vi "tx poulse host.vi"() -> ()   [LabVIEW 2021]
uses:
  random_limits.ctl
  emitter params.ctl
  mode_type.ctl
  <vilib>/userdefined/High Color/nirio_resource_hc.ctl
  secnario config.ctl
  <instrlib>/niUsrpRio/Config/v1/Host/Public/niUsrpRio Session.ctl
  <instrlib>/_niInstr/Register Bus/v0/Host/Public/Register Bus Session.ctl
  <instrlib>/_niInstr/Register Bus/v0/Host/Private/Session Data.ctl
  <instrlib>/niUsrpRio/Config/v1/Host/Private/DB Queue Reference.ctl
  <instrlib>/niUsrpRio/Config/v1/Host/Private/Daughterboard Data.ctl
  <instrlib>/niUsrpRio/Config/v1/Host/Private/ATR state data.ctl
  <instrlib>/niUsrpRio/Config/v1/Host/Private/Antenna Configuration.ctl
  <instrlib>/niUsrpRio/Config/v1/Host/Private/CPLD Power Mode.ctl
  <instrlib>/niUsrpRio/Config/v1/Host/Public/EEPROM Header.ctl
  <instrlib>/niUsrpRio/Config/v1/Host/Public/EEPROM Device Data Header.ctl
  <instrlib>/niUsrpRio/Config/v1/Host/Public/EEPROM Characterization Header.ctl
  <instrlib>/niUsrpRio/Config/v1/Host/Public/Characterization Data.ctl
  <instrlib>/niUsrpRio/Config/v1/Host/Public/IQ Imbalance.ctl
  <instrlib>/_niInstr/Register Bus/v0/Host/niInstr Register Bus v0 Host.lvlib
  <instrlib>/niUsrpRio/Config/v1/Host/niUsrpRio Config v1 Host.lvlib
panel:
  in  "end program":bool
  in  "Tab Control":T1(tab)=enum."tx configuration"
  in  "user configurations":T3={"vst_device"=["VST_1", "VST_2"], "file paths"=[path "C:/Users/PXIe8108_Demo/Documents/CHAIM DATA/chaim/5785_sync_for_elbit/data/pdw_test_file.tdms", path "C:/Users/PXIe8108_Demo/Documents/CHAIM DATA/chaim/5785_sync_for_elbit/data/pdw_test_file_1.tdms", path "C:/Users/PXIe8108_Demo/Documents/CHAIM DATA/chaim/5785_sync_for_elbit/data/pdw_test_file_2.tdms", path "C:/Users/PXIe8108_Demo/Documents/CHAIM DATA/chaim/5785_sync_for_elbit/data/pdw_test_file_3.tdms", path "C:/Users/PXIe8108_Demo/Documents/CHAIM DATA/chaim/5785_sync_for_elbit/data/pdw_test_file_4.tdms"], "RF gain "=10.0, "devicess "=["IF_transiver_0", "IF_transiver_1", "IF_transiver_2"], "buffer size"=524288, "center frequency (Hz) "=1000000000.0, "Dial"=1, "P2P sample rate"=200000000.0} {"P2P sample rate" format="%#.8p"; "Dial" scale=0.0..3.0; "center frequency (Hz)" format="%#.8p"; "buffer size" step=512; "RF gain" min=-130.0 max=30.0 format="%#.8p"}
  in  "generate":bool
  in  "Tab Control 2":T4(tab)
  in  "rand limits":T5={"DOA range "={1634128.9560392164, 2964508.639841233}, "modulation depth"={67532.40039072247, 205475.5312375231}, "num of hoopers"=25, "num of frequncyes"={2, 1}, "QPSK"=TRUE, "BPSK"=TRUE, "LFM"=TRUE, "CW"=TRUE, "     f band range"={903686635.9447005, 1095391705.0691245}, "D.C range"={0.09831029185867896, 0.026113671274961597}, "hop rate range"={2.0915680786684536, 1602.2122593840786}, "span range "={1634128.9560392164, 2964508.639841233}, "amp range"={-21.121351766513058, -25.88325652841782}, "start time (sec)"=0.0, "end time (sec)"=50.0} {"start time (sec)" format="%#_13g"; "amp range" scale=0.0..-50.0 scale format="%#_g dB"; "span range" scale=1000000.0..3000000000.0 scale format="%#_6p Hz"; "hop rate range" scale=1.0..3000.0 scale format="%#_6p"; "D.C range" scale=0.0..1.0; "f band range" scale=920000000.0..1080000000.0 scale format="%#_6p Hz"; "num of frequncyes" scale=1.0..300.0; "num of hoopers" scale=0.0..200.0; "modulation depth" scale=10000.0..30000000.0 scale format="%#_6p Hz"; "DOA range" scale=0.0..360.0 scale format="%#_6p deg"}
  in  "user bulid emitters":T6[](array[typedef]) {"t end" format="%#_3p"; "t start" format="%#_3p"; "DOA" format="%#_3p"; "mod depth" format="%.0p"}
  in  "convert Button":bool
  in  "csv pulse istraction file in":path=path "C:/Users/PXIe8108_Demo/Documents/CHAIM DATA/chaim/5785_sync_for_elbit/data/pdw_test_file_1.tdms"
  in  "gen for DF":bool=TRUE
  out "num of pulses":i32=902603
  in  "color plate":T8={"PSK Color"=4591, "LFM Color"=15663139, "CW Color"=0}
  in  "refresh_file show":bool
  in  "max number of pulses to show":dbl=500.0
  in  "time range":cluster{dbl, dbl}(slide)={0.0, 78525345.62211981} scale=0.0..50.0 scale format="%#_6p sec"
  out "XY Graph":cluster{dbl[], dbl[]}[](graph)=[{[995507474.9163239, 995507474.9163239, 995394224.6331983, 995394224.6331983, 995507474.9163239], [1.3135e-05, 6.3885e-05, 6.3885e-05, 1.3135e-05, 1.3135e-05]}, {[988830819.370068, 988830819.370068, 988758224.0887612, 988758224.0887612, 988830819.370068], [4.3525e-05, 9.444999999999999e-05, 9.444999999999999e-05, 4.3525e-05, 4.3525e-05]}, {[1062189174.9203769, 1062189174.9203769], [0.000208895, 0.00027960500000000004]}, {[929162452.3956556, 929162452.3956556], [0.00021476, 0.000257185]}, {[1021330874.2578875, 1021330874.2578875], [0.000356845, 0.00040845]}, {[1073135024.1335804, 1073135024.1335804], [0.000418565, 0.000526315]}, {[1060251782.7954887, 1060251782.7954887, 1060128932.6726385, 1060128932.6726385, 1060251782.7954887], [0.000515485, 0.00053533, 0.00053533, 0.000515485, 0.000515485]}, {[1026728042.2238628, 1026728042.2238628], [0.000518575, 0.000544775]}, {[984517369.6351253, 984599401.9622253], [0.000526025, 0.000625825]}, {[992027316.0868192, 992176780.8711365], [0.000643445, 0.00067611]}, {[928917483.6448978, 929054857.2098373], [0.0007013, 0.0007404499999999999]}, {[989419092.0700991, 989419092.0700991, 989346496.7887924, 989346496.7887924, 989419092.0700991], [0.000739625, 0.00079055, 0.00079055, 0.000739625, 0.000739625]}, {[1054560346.3581073, 1054742969.627864], [0.000739975, 0.00084052]}, {[1082291065.6729505, 1082469758.1538203], [0.000779595, 0.00084535]}, {[1050818739.1925838, 1050818739.1925838, 1050641119.2991557, 1050641119.2991557, 1050818739.1925838], [0.000827985, 0.000929745, 0.000929745, 0.000827985, 0.000827985]}, {[1067340749.8623314, 1067340749.8623314, 1067233912.2554936, 1067233912.2554936, 1067340749.8623314], [0.000864145, 0.000954195, 0.000954195, 0.000864145, 0.000864145]}, {[929162452.3956556, 929162452.3956556], [0.001105885, 0.00114831]}, {[996643673.8301789, 996643673.8301789, 996530423.5470532, 996530423.5470532, 996643673.8301789], [0.00112341, 0.00117416, 0.00117416, 0.00112341, 0.00112341]}, {[1082864717.4175386, 1082864717.4175386, 1082774950.8107162, 1082774950.8107162, 1082864717.4175386], [0.001128215, 0.0014517599999999999, 0.0014517599999999999, 0.001128215, 0.001128215]}, {[1031645785.7104015, 1031645785.7104015, 1031564879.5615342, 1031564879.5615342, 1031645785.7104015], [0.00115809, 0.0016224, 0.0016224, 0.00115809, 0.00115809]}, {[1020995471.866172, 1020995471.866172], [0.00117441, 0.001226015]}, {[1062189174.9203769, 1062189174.9203769], [0.001185005, 0.0012557150000000001]}, {[1060210906.3844512, 1060210906.3844512, 1060088056.261601, 1060088056.261601, 1060210906.3844512], [0.001244975, 0.00126482, 0.00126482, 0.001244975, 0.001244975]}, {[1026728042.2238628, 1026728042.2238628], [0.001275565, 0.001301765]}, {[994154871.3947781, 994304336.1790955], [0.00136976, 0.0014024250000000001]}, {[1060103621.4849387, 1060103621.4849387], [0.001372985, 0.0014659949999999999]}, {[988830819.370068, 988830819.370068, 988758224.0887612, 988758224.0887612, 988830819.370068], [0.001435725, 0.00148665, 0.00148665, 0.001435725, 0.001435725]}, {[927476484.2448008, 927613857.8097403], [0.00145419, 0.00149334]}, {[907652360.3992398, 907652360.3992398, 907562914.960957, 907562914.960957, 907652360.3992398], [0.001505205, 0.001655765, 0.001655765, 0.001505205, 0.001505205]}, {[1010524208.2116058, 1010524208.2116058, 1010446688.8317609, 1010446688.8317609, 1010524208.2116058], [0.001643815, 0.0022050100000000003, 0.0022050100000000003, 0.001643815, 0.001643815]}, {[1027479006.2384171, 1027479006.2384171, 1027398361.0771267, 1027398361.0771267, 1027479006.2384171], [0.001671275, 0.0017460800000000001, 0.0017460800000000001, 0.001671275, 0.001671275]}, {[1073152530.0637031, 1073152530.0637031], [0.001702195, 0.001809945]}, {[1080469326.322043, 1080648018.8029127], [0.00176813, 0.001833885]}, {[984517369.6351253, 984599401.9622253], [0.001798725, 0.0018985249999999999]}, {[1055565518.0981148, 1055748141.3678715], [0.001900405, 0.00200095]}, {[1060251782.7954887, 1060251782.7954887, 1060128932.6726385, 1060128932.6726385, 1060251782.7954887], [0.00197447, 0.001994315, 0.001994315, 0.00197447, 0.00197447]}, {[1021330874.2578875, 1021330874.2578875], [0.001991975, 0.00204358]}, {[929162452.3956556, 929162452.3956556], [0.001997015, 0.00203944]}, {[1026728042.2238628, 1026728042.2238628], [0.00203255, 0.0020587500000000002]}, {[992027316.0868192, 992176780.8711365], [0.00209608, 0.002128745]}, {[989419092.0700991, 989419092.0700991, 989346496.7887924, 989346496.7887924, 989419092.0700991], [0.002131825, 0.00218275, 0.00218275, 0.002131825, 0.002131825]}, {[1062189174.9203769, 1062189174.9203769], [0.00216112, 0.0022318299999999998]}, {[928917483.6448978, 929054857.2098373], [0.00220708, 0.00224623]}, {[995507474.9163239, 995507474.9163239, 995394224.6331983, 995394224.6331983, 995507474.9163239], [0.002233685, 0.002284435, 0.002284435, 0.002233685, 0.002233685]}, {[1051290310.7105097, 1051290310.7105097, 1051112690.8170816, 1051112690.8170816, 1051290310.7105097], [0.00251469, 0.00261645, 0.00261645, 0.00251469, 0.00251469]}, {[1060210906.3844512, 1060210906.3844512, 1060088056.261601, 1060088056.261601, 1060210906.3844512], [0.00270396, 0.002723805, 0.002723805, 0.00270396, 0.00270396]}, {[1082291065.6729505, 1082469758.1538203], [0.00275667, 0.002822425]}, {[1026728042.2238628, 1026728042.2238628], [0.00278954, 0.00281574]}, {[1067340749.8623314, 1067340749.8623314, 1067233912.2554936, 1067233912.2554936, 1067340749.8623314], [0.002802505, 0.0028925549999999998, 0.0028925549999999998, 0.002802505, 0.002802505]}, {[1020995471.866172, 1020995471.866172], [0.002809545, 0.0028611500000000002]}, {[994154871.3947781, 994304336.1790955], [0.002822395, 0.00285506]}, {[988830819.370068, 988830819.370068, 988758224.0887612, 988758224.0887612, 988830819.370068], [0.002827925, 0.0028788499999999996, 0.0028788499999999996, 0.002827925, 0.002827925]}, {[929162452.3956556, 929162452.3956556], [0.00288814, 0.002930565]}, {[927476484.2448008, 927613857.8097403], [0.002959975, 0.002999125]}, {[1073135024.1335804, 1073135024.1335804], [0.00298583, 0.0030935800000000003]}, {[1054560346.3581073, 1054742969.627864], [0.00306084, 0.003161385]}, {[984517369.6351253, 984599401.9622253], [0.003071425, 0.003171225]}, {[1062189174.9203769, 1062189174.9203769], [0.00313723, 0.00320794]}, {[959254135.8898987, 959254135.8898987, 959109313.2975742, 959109313.2975742, 959254135.8898987], [0.00317855, 0.00356861, 0.00356861, 0.00317855, 0.00317855]}, {[996643673.8301789, 996643673.8301789, 996530423.5470532, 996530423.5470532, 996643673.8301789], [0.00334396, 0.00339471, 0.00339471, 0.00334396, 0.00334396]}, {[1060251782.7954887, 1060251782.7954887, 1060128932.6726385, 1060128932.6726385, 1060251782.7954887], [0.00343345, 0.003453295, 0.003453295, 0.00343345, 0.00343345]}, {[989419092.0700991, 989419092.0700991, 989346496.7887924, 989346496.7887924, 989419092.0700991], [0.00352402, 0.003574945, 0.003574945, 0.00352402, 0.00352402]}, {[1026728042.2238628, 1026728042.2238628], [0.003546525, 0.003572725]}, {[992027316.0868192, 992176780.8711365], [0.00354871, 0.003581375]}, {[1021330874.2578875, 1021330874.2578875], [0.00362711, 0.003678715]}, {[909232485.1651794, 909232485.1651794, 909143039.7268966, 909143039.7268966, 909232485.1651794], [0.00371271, 0.0038632700000000002, 0.0038632700000000002, 0.00371271, 0.00371271]}, {[928917483.6448978, 929054857.2098373], [0.003712865, 0.003752015]}, {[1080469326.322043, 1080648018.8029127], [0.00374521, 0.003810965]}, {[929162452.3956556, 929162452.3956556], [0.00377927, 0.003821695]}, {[1060103621.4849387, 1060103621.4849387], [0.00394052, 0.0040335300000000004]}, {[1062189174.9203769, 1062189174.9203769], [0.004113345, 0.004184055]}, {[1028479722.7550542, 1028479722.7550542, 1028399077.5937638, 1028399077.5937638, 1028479722.7550542], [0.004155185, 0.0042299899999999994, 0.0042299899999999994, 0.004155185, 0.004155185]}, {[1060210906.3844512, 1060210906.3844512, 1060088056.261601, 1060088056.261601, 1060210906.3844512], [0.00416294, 0.0041827850000000005, 0.0041827850000000005, 0.00416294, 0.00416294]}, {[1050818739.1925838, 1050818739.1925838, 1050641119.2991557, 1050641119.2991557, 1050818739.1925838], [0.00420139, 0.00430315, 0.00430315, 0.00420139, 0.00420139]}, {[988830819.370068, 988830819.370068, 988758224.0887612, 988758224.0887612, 988830819.370068], [0.00422012, 0.004271045, 0.004271045, 0.00422012, 0.00422012]}, {[1055565518.0981148, 1055748141.3678715], [0.00422127, 0.004321815]}, {[1073152530.0637031, 1073152530.0637031], [0.00426946, 0.00437721]}, {[994154871.3947781, 994304336.1790955], [0.00427503, 0.004307695]}, {[1026728042.2238628, 1026728042.2238628], [0.004303515, 0.004329715]}, {[984517369.6351253, 984599401.9622253], [0.004344125, 0.004443925]}, {[1020995471.866172, 1020995471.866172], [0.004444675, 0.00449628]}, {[995507474.9163239, 995507474.9163239, 995394224.6331983, 995394224.6331983, 995507474.9163239], [0.004454235, 0.0045049849999999995, 0.0045049849999999995, 0.004454235, 0.004454235]}, {[927476484.2448008, 927613857.8097403], [0.004465755, 0.004504905]}, {[929162452.3956556, 929162452.3956556], [0.004670395, 0.0047128199999999995]}, {[1083149040.2114863, 1083149040.2114863, 1083059273.6046643, 1083059273.6046643, 1083149040.2114863], [0.00472927, 0.0050528149999999996, 0.0050528149999999996, 0.00472927, 0.00472927]}, {[1082291065.6729505, 1082469758.1538203], [0.004733745, 0.0047995]}, {[1067340749.8623314, 1067340749.8623314, 1067233912.2554936, 1067233912.2554936, 1067340749.8623314], [0.00474086, 0.004830910000000001, 0.004830910000000001, 0.00474086, 0.00474086]}, {[1060251782.7954887, 1060251782.7954887, 1060128932.6726385, 1060128932.6726385, 1060251782.7954887], [0.004892435, 0.00491228, 0.00491228, 0.004892435, 0.004892435]}, {[989419092.0700991, 989419092.0700991, 989346496.7887924, 989346496.7887924, 989419092.0700991], [0.00491622, 0.004967145, 0.004967145, 0.00491622, 0.00491622]}, {[992027316.0868192, 992176780.8711365], [0.005001345, 0.00503401]}, {[1026728042.2238628, 1026728042.2238628], [0.0050605, 0.0050866999999999996]}, {[1062189174.9203769, 1062189174.9203769], [0.005089455, 0.0051601649999999995]}, {[928917483.6448978, 929054857.2098373], [0.005218645, 0.005257795]}, {[958900541.628188, 958900541.628188, 958736338.0157086, 958736338.0157086, 958900541.628188], [0.00525029, 0.00584843, 0.00584843, 0.00525029, 0.00525029]}, {[1021330874.2578875, 1021330874.2578875], [0.00526224, 0.005313844999999999]}, {[1054560346.3581073, 1054742969.627864], [0.005381705, 0.005482249999999999]}, {[1073135024.1335804, 1073135024.1335804], [0.005553095, 0.005660845]}, {[929162452.3956556, 929162452.3956556], [0.00556152, 0.005603945]}, {[996643673.8301789, 996643673.8301789, 996530423.5470532, 996530423.5470532, 996643673.8301789], [0.005564505, 0.0056152549999999996, 0.0056152549999999996, 0.005564505, 0.005564505]}, {[988830819.370068, 988830819.370068, 988758224.0887612, 988758224.0887612, 988830819.370068], [0.00561232, 0.005663245, 0.005663245, 0.00561232, 0.00561232]}, {[984517369.6351253, 984599401.9622253], [0.005616825, 0.0057166249999999995]}, {[1060210906.3844512, 1060210906.3844512, 1060088056.261601, 1060088056.261601, 1060210906.3844512], [0.005621925, 0.00564177, 0.00564177, 0.005621925, 0.005621925]}, {[1080469326.322043, 1080648018.8029127], [0.005722285, 0.0057880399999999995]}, {[994154871.3947781, 994304336.1790955], [0.00572766, 0.005760325]}, {[1026728042.2238628, 1026728042.2238628], [0.00581749, 0.0058436899999999995]}, {[1051290310.7105097, 1051290310.7105097, 1051112690.8170816, 1051112690.8170816, 1051290310.7105097], [0.005888095, 0.0059898550000000005, 0.0059898550000000005, 0.005888095, 0.005888095]}, {[907652360.3992398, 907652360.3992398, 907562914.960957, 907562914.960957, 907652360.3992398], [0.005920215, 0.0060707750000000005, 0.0060707750000000005, 0.005920215, 0.005920215]}, {[927476484.2448008, 927613857.8097403], [0.005971535, 0.006010685]}, {[1062189174.9203769, 1062189174.9203769], [0.00606557, 0.00613628]}, {[1020995471.866172, 1020995471.866172], [0.00607981, 0.0061314149999999994]}, {[989419092.0700991, 989419092.0700991, 989346496.7887924, 989346496.7887924, 989419092.0700991], [0.006308415, 0.006359340000000001, 0.006359340000000001, 0.006308415, 0.006308415]}, {[1060251782.7954887, 1060251782.7954887, 1060128932.6726385, 1060128932.6726385, 1060251782.7954887], [0.006351415, 0.00637126, 0.00637126, 0.006351415, 0.006351415]}, {[1032360862.9064839, 1032360862.9064839, 1032279956.7576165, 1032279956.7576165, 1032360862.9064839], [0.006364295, 0.006828605, 0.006828605, 0.006364295, 0.006364295]}, {[929162452.3956556, 929162452.3956556], [0.00645265, 0.0064950749999999995]}, {[992027316.0868192, 992176780.8711365], [0.00645398, 0.006486645]}, {[1060103621.4849387, 1060103621.4849387], [0.00650806, 0.0066010700000000005]}, {[1055565518.0981148, 1055748141.3678715], [0.006542135, 0.00664268]}, {[1026728042.2238628, 1026728042.2238628], [0.00657448, 0.006600679999999999]}, {[1027479006.2384171, 1027479006.2384171, 1027398361.0771267, 1027398361.0771267, 1027479006.2384171], [0.006639095, 0.0067139, 0.0067139, 0.006639095, 0.006639095]}, {[995507474.9163239, 995507474.9163239, 995394224.6331983, 995394224.6331983, 995507474.9163239], [0.00667478, 0.0067255299999999995, 0.0067255299999999995, 0.00667478, 0.00667478]}, {[1067340749.8623314, 1067340749.8623314, 1067233912.2554936, 1067233912.2554936, 1067340749.8623314], [0.00667922, 0.00676927, 0.00676927, 0.00667922, 0.00667922]}, {[1082291065.6729505, 1082469758.1538203], [0.006710825, 0.00677658]}, {[928917483.6448978, 929054857.2098373], [0.006724425, 0.006763575]}, {[1073152530.0637031, 1073152530.0637031], [0.00683673, 0.00694448]}, {[984517369.6351253, 984599401.9622253], [0.006889525, 0.006989324999999999]}, {[1021330874.2578875, 1021330874.2578875], [0.006897375, 0.00694898]}, {[988830819.370068, 988830819.370068, 988758224.0887612, 988758224.0887612, 988830819.370068], [0.007004515, 0.0070554400000000005, 0.0070554400000000005, 0.007004515, 0.007004515]}, {[1062189174.9203769, 1062189174.9203769], [0.00704168, 0.00711239]}, {[1060210906.3844512, 1060210906.3844512, 1060088056.261601, 1060088056.261601, 1060210906.3844512], [0.007080905, 0.00710075, 0.00710075, 0.007080905, 0.007080905]}, {[994154871.3947781, 994304336.1790955], [0.007180295, 0.00721296]}, {[1026728042.2238628, 1026728042.2238628], [0.007331465, 0.007357664999999999]}, {[929162452.3956556, 929162452.3956556], [0.007343775, 0.0073862]}, {[927476484.2448008, 927613857.8097403], [0.00747732, 0.00751647]}, {[1050818739.1925838, 1050818739.1925838, 1050641119.2991557, 1050641119.2991557, 1050818739.1925838], [0.0075748, 0.00767656, 0.00767656, 0.0075748, 0.0075748]}, {[959254135.8898987, 959254135.8898987, 959109313.2975742, 959109313.2975742, 959254135.8898987], [0.00769425, 0.008084309999999999, 0.008084309999999999, 0.00769425, 0.00769425]}, {[1080469326.322043, 1080648018.8029127], [0.00769936, 0.0077651149999999995]}, {[989419092.0700991, 989419092.0700991, 989346496.7887924, 989346496.7887924, 989419092.0700991], [0.007700615, 0.00775154, 0.00775154, 0.007700615, 0.007700615]}, {[1054560346.3581073, 1054742969.627864], [0.00770257, 0.007803114999999999]}, {[1020995471.866172, 1020995471.866172], [0.00771494, 0.007766545]}, {[996643673.8301789, 996643673.8301789, 996530423.5470532, 996530423.5470532, 996643673.8301789], [0.007785055, 0.007835805, 0.007835805, 0.007785055, 0.007785055]}, {[1060251782.7954887, 1060251782.7954887, 1060128932.6726385, 1060128932.6726385, 1060251782.7954887], [0.0078104, 0.007830245, 0.007830245, 0.0078104, 0.0078104]}, {[992027316.0868192, 992176780.8711365], [0.00790661, 0.007939274999999999]}, {[1062189174.9203769, 1062189174.9203769], [0.008017795, 0.008088505]}, {[1010524208.2116058, 1010524208.2116058, 1010446688.8317609, 1010446688.8317609, 1010524208.2116058], [0.008022065, 0.00858326, 0.00858326, 0.008022065, 0.008022065]}, {[1026728042.2238628, 1026728042.2238628], [0.008088455, 0.008114655]}, {[1073135024.1335804, 1073135024.1335804], [0.00812036, 0.00822811]}, {[909232485.1651794, 909232485.1651794, 909143039.7268966, 909143039.7268966, 909232485.1651794], [0.00812772, 0.008278279999999999, 0.008278279999999999, 0.00812772, 0.00812772]}, {[984517369.6351253, 984599401.9622253], [0.008162225, 0.008262025000000001]}, {[928917483.6448978, 929054857.2098373], [0.00823021, 0.00826936]}, {[929162452.3956556, 929162452.3956556], [0.0082349, 0.008277325]}, {[1082864717.4175386, 1082864717.4175386, 1082774950.8107162, 1082774950.8107162, 1082864717.4175386], [0.00833032, 0.008653865, 0.008653865, 0.00833032, 0.00833032]}, {[988830819.370068, 988830819.370068, 988758224.0887612, 988758224.0887612, 988830819.370068], [0.008396715, 0.008447640000000001, 0.008447640000000001, 0.008396715, 0.008396715]}, {[1021330874.2578875, 1021330874.2578875], [0.008532505, 0.008584109999999999]}, {[1060210906.3844512, 1060210906.3844512, 1060088056.261601, 1060088056.261601, 1060210906.3844512], [0.00853989, 0.008559734999999999, 0.008559734999999999, 0.00853989, 0.00853989]}, {[1067340749.8623314, 1067340749.8623314, 1067233912.2554936, 1067233912.2554936, 1067340749.8623314], [0.00861758, 0.00870763, 0.00870763, 0.00861758, 0.00861758]}, {[994154871.3947781, 994304336.1790955], [0.00863293, 0.008665595]}, {[1082291065.6729505, 1082469758.1538203], [0.0086879, 0.008753655]}, {[1026728042.2238628, 1026728042.2238628], [0.00884544, 0.00887164]}, {[1055565518.0981148, 1055748141.3678715], [0.008863, 0.008963545]}, {[1071939451.6053249, 1071939451.6053249, 1071769816.3211857, 1071769816.3211857, 1071939451.6053249], [0.008890785, 0.009210155, 0.009210155, 0.008890785, 0.008890785]}, {[995507474.9163239, 995507474.9163239, 995394224.6331983, 995394224.6331983, 995507474.9163239], [0.00889533, 0.00894608, 0.00894608, 0.00889533, 0.00889533]}, {[920932748.9465165, 920932748.9465165, 920784710.4565091, 920784710.4565091, 920932748.9465165], [0.00893469, 0.009550165000000001, 0.009550165000000001, 0.00893469, 0.00893469]}, {[927476484.2448008, 927613857.8097403], [0.0089831, 0.00902225]}, {[1062189174.9203769, 1062189174.9203769], [0.008993905, 0.009064615]}, {[1060103621.4849387, 1060103621.4849387], [0.009075595, 0.009168605]}, {[989419092.0700991, 989419092.0700991, 989346496.7887924, 989346496.7887924, 989419092.0700991], [0.009092815, 0.009143740000000001, 0.009143740000000001, 0.009092815, 0.009092815]}, {[1028479722.7550542, 1028479722.7550542, 1028399077.5937638, 1028399077.5937638, 1028479722.7550542], [0.009123005, 0.00919781, 0.00919781, 0.009123005, 0.009123005]}, {[929162452.3956556, 929162452.3956556], [0.00912603, 0.009168455]}, {[1051290310.7105097, 1051290310.7105097, 1051112690.8170816, 1051112690.8170816, 1051290310.7105097], [0.009261505, 0.009363264999999999, 0.009363264999999999, 0.009261505, 0.009261505]}, {[1060251782.7954887, 1060251782.7954887, 1060128932.6726385, 1060128932.6726385, 1060251782.7954887], [0.00926938, 0.009289225, 0.009289225, 0.00926938, 0.00926938]}, {[1020995471.866172, 1020995471.866172], [0.009350075, 0.009401679999999999]}, {[992027316.0868192, 992176780.8711365], [0.009359245, 0.00939191]}, {[1073152530.0637031, 1073152530.0637031], [0.009403995, 0.009511745]}, {[984517369.6351253, 984599401.9622253], [0.009434925, 0.009534725]}, {[1026728042.2238628, 1026728042.2238628], [0.00960243, 0.009628630000000001]}, {[1080469326.322043, 1080648018.8029127], [0.009676435, 0.009742190000000001]}, {[928917483.6448978, 929054857.2098373], [0.00973599, 0.00977514]}, {[988830819.370068, 988830819.370068, 988758224.0887612, 988758224.0887612, 988830819.370068], [0.00978891, 0.009839835, 0.009839835, 0.00978891, 0.00978891]}, {[1062189174.9203769, 1062189174.9203769], [0.00997002, 0.01004073]}, {[1060210906.3844512, 1060210906.3844512, 1060088056.261601, 1060088056.261601, 1060210906.3844512], [0.00999887, 0.010018715, 0.010018715, 0.00999887, 0.00999887]}, {[996643673.8301789, 996643673.8301789, 996530423.5470532, 996530423.5470532, 996643673.8301789], [0.010005605, 0.010056355000000001, 0.010056355000000001, 0.010005605, 0.010005605]}, {[929162452.3956556, 929162452.3956556], [0.010017155, 0.01005958]}, {[1054560346.3581073, 1054742969.627864], [0.010023435, 0.010123980000000001]}, {[994154871.3947781, 994304336.1790955], [0.01008556, 0.010118225]}, {[1021330874.2578875, 1021330874.2578875], [0.01016764, 0.010219245]}, {[907652360.3992398, 907652360.3992398, 907562914.960957, 907562914.960957, 907652360.3992398], [0.010335225, 0.010485785, 0.010485785, 0.010335225, 0.010335225]}, {[1026728042.2238628, 1026728042.2238628], [0.010359415, 0.010385615]}, {[989419092.0700991, 989419092.0700991, 989346496.7887924, 989346496.7887924, 989419092.0700991], [0.01048501, 0.010535935, 0.010535935, 0.01048501, 0.01048501]}, {[927476484.2448008, 927613857.8097403], [0.01048888, 0.01052803]}, {[1067340749.8623314, 1067340749.8623314, 1067233912.2554936, 1067233912.2554936, 1067340749.8623314], [0.010555935, 0.010645985, 0.010645985, 0.010555935, 0.010555935]}, {[1082291065.6729505, 1082469758.1538203], [0.010664975, 0.01073073]}, {[1073135024.1335804, 1073135024.1335804], [0.010687625, 0.010795375]}, {[984517369.6351253, 984599401.9622253], [0.010707625, 0.010807425]}, {[1060251782.7954887, 1060251782.7954887, 1060128932.6726385, 1060128932.6726385, 1060251782.7954887], [0.01072836, 0.010748204999999999, 0.010748204999999999, 0.01072836, 0.01072836]}, {[992027316.0868192, 992176780.8711365], [0.01081188, 0.010844544999999999]}, {[929162452.3956556, 929162452.3956556], [0.01090828, 0.010950705]}, {[1062189174.9203769, 1062189174.9203769], [0.01094613, 0.01101684]}, {[1050818739.1925838, 1050818739.1925838, 1050641119.2991557, 1050641119.2991557, 1050818739.1925838], [0.01094821, 0.01104997, 0.01104997, 0.01094821, 0.01094821]}, {[1020995471.866172, 1020995471.866172], [0.010985205, 0.01103681]}, {[995507474.9163239, 995507474.9163239, 995394224.6331983, 995394224.6331983, 995507474.9163239], [0.01111588, 0.01116663, 0.01116663, 0.01111588, 0.01111588]}, {[1026728042.2238628, 1026728042.2238628], [0.011116405, 0.011142605]}, {[988830819.370068, 988830819.370068, 988758224.0887612, 988758224.0887612, 988830819.370068], [0.01118111, 0.011232035, 0.011232035, 0.01118111, 0.01118111]}, {[1055565518.0981148, 1055748141.3678715], [0.011183865, 0.01128441]}, {[928917483.6448978, 929054857.2098373], [0.011241775, 0.011280925]}, {[1060210906.3844512, 1060210906.3844512, 1060088056.261601, 1060088056.261601, 1060210906.3844512], [0.011457855, 0.011477699999999999, 0.011477699999999999, 0.011457855, 0.011457855]}, {[994154871.3947781, 994304336.1790955], [0.011538195, 0.011570859999999999]}, {[1031645785.7104015, 1031645785.7104015, 1031564879.5615342, 1031564879.5615342, 1031645785.7104015], [0.011570505, 0.012034815, 0.012034815, 0.011570505, 0.011570505]}, {[1027479006.2384171, 1027479006.2384171, 1027398361.0771267, 1027398361.0771267, 1027479006.2384171], [0.011606915, 0.011681720000000001, 0.011681720000000001, 0.011606915, 0.011606915]}, {[1060103621.4849387, 1060103621.4849387], [0.01164313, 0.011736139999999999]}, {[1080469326.322043, 1080648018.8029127], [0.011653515, 0.01171927]}, {[929162452.3956556, 929162452.3956556], [0.01179941, 0.011841835]}, {[1021330874.2578875, 1021330874.2578875], [0.01180277, 0.011854375]}, {[1026728042.2238628, 1026728042.2238628], [0.011873395, 0.011899595]}, {[989419092.0700991, 989419092.0700991, 989346496.7887924, 989346496.7887924, 989419092.0700991], [0.01187721, 0.011928135, 0.011928135, 0.01187721, 0.01187721]}, {[1062189174.9203769, 1062189174.9203769], [0.011922245, 0.011992955]}, {[1083149040.2114863, 1083149040.2114863, 1083059273.6046643, 1083059273.6046643, 1083149040.2114863], [0.01193137, 0.012254915, 0.012254915, 0.01193137, 0.01193137]}, {[1073152530.0637031, 1073152530.0637031], [0.01197126, 0.01207901]}, {[984517369.6351253, 984599401.9622253], [0.011980325, 0.012080125]}, {[927476484.2448008, 927613857.8097403], [0.011994665, 0.012033815]}, {[1060251782.7954887, 1060251782.7954887, 1060128932.6726385, 1060128932.6726385, 1060251782.7954887], [0.012187345, 0.01220719, 0.01220719, 0.012187345, 0.012187345]}, {[959254135.8898987, 959254135.8898987, 959109313.2975742, 959109313.2975742, 959254135.8898987], [0.01220995, 0.01260001, 0.01260001, 0.01220995, 0.01220995]}, {[996643673.8301789, 996643673.8301789, 996530423.5470532, 996530423.5470532, 996643673.8301789], [0.01222615, 0.0122769, 0.0122769, 0.01222615, 0.01222615]}, {[992027316.0868192, 992176780.8711365], [0.01226451, 0.012297174999999999]}, {[1054560346.3581073, 1054742969.627864], [0.012344295, 0.01244484]}, {[1067340749.8623314, 1067340749.8623314, 1067233912.2554936, 1067233912.2554936, 1067340749.8623314], [0.012494295, 0.012584345, 0.012584345, 0.012494295, 0.012494295]}, {[909232485.1651794, 909232485.1651794, 909143039.7268966, 909143039.7268966, 909232485.1651794], [0.01254273, 0.01269329, 0.01269329, 0.01254273, 0.01254273]}, {[988830819.370068, 988830819.370068, 988758224.0887612, 988758224.0887612, 988830819.370068], [0.01257331, 0.012624235000000001, 0.012624235000000001, 0.01257331, 0.01257331]}, {[1020995471.866172, 1020995471.866172], [0.01262034, 0.012671945]}, {[1026728042.2238628, 1026728042.2238628], [0.01263038, 0.01265658]}, {[1051290310.7105097, 1051290310.7105097, 1051112690.8170816, 1051112690.8170816, 1051290310.7105097], [0.01263491, 0.012736669999999999, 0.012736669999999999, 0.01263491, 0.01263491]}, {[1082291065.6729505, 1082469758.1538203], [0.01264205, 0.012707805]}, {[929162452.3956556, 929162452.3956556], [0.012690535, 0.01273296]}, {[928917483.6448978, 929054857.2098373], [0.012747555, 0.012786705]}, {[1062189174.9203769, 1062189174.9203769], [0.012898355, 0.012969065]}, {[1060210906.3844512, 1060210906.3844512, 1060088056.261601, 1060088056.261601, 1060210906.3844512], [0.012916835, 0.012936679999999999, 0.012936679999999999, 0.012916835, 0.012916835]}, {[958900541.628188, 958900541.628188, 958736338.0157086, 958736338.0157086, 958900541.628188], [0.01294312, 0.013541260000000001, 0.013541260000000001, 0.01294312, 0.01294312]}, {[994154871.3947781, 994304336.1790955], [0.01299083, 0.013023495]}, {[984517369.6351253, 984599401.9622253], [0.013253025, 0.013352825]}, {[1073135024.1335804, 1073135024.1335804], [0.01325489, 0.01336264]}, {[989419092.0700991, 989419092.0700991, 989346496.7887924, 989346496.7887924, 989419092.0700991], [0.013269405, 0.01332033, 0.01332033, 0.013269405, 0.013269405]}, {[995507474.9163239, 995507474.9163239, 995394224.6331983, 995394224.6331983, 995507474.9163239], [0.013336425, 0.013387175000000001, 0.013387175000000001, 0.013336425, 0.013336425]}, {[1026728042.2238628, 1026728042.2238628], [0.01338737, 0.013413570000000001]}, {[1021330874.2578875, 1021330874.2578875], [0.013437905, 0.01348951]}, {[927476484.2448008, 927613857.8097403], [0.013500445, 0.013539595]}, {[1055565518.0981148, 1055748141.3678715], [0.01350473, 0.013605275]}, {[929162452.3956556, 929162452.3956556], [0.013581665, 0.01362409]}, {[1080469326.322043, 1080648018.8029127], [0.01363059, 0.013696345]}, {[1060251782.7954887, 1060251782.7954887, 1060128932.6726385, 1060128932.6726385, 1060251782.7954887], [0.013646325, 0.01366617, 0.01366617, 0.013646325, 0.013646325]}, {[992027316.0868192, 992176780.8711365], [0.013717145, 0.01374981]}, {[1062189174.9203769, 1062189174.9203769], [0.01387447, 0.01394518]}, {[988830819.370068, 988830819.370068, 988758224.0887612, 988758224.0887612, 988830819.370068], [0.013965505, 0.01401643, 0.01401643, 0.013965505, 0.013965505]}, {[1028479722.7550542, 1028479722.7550542, 1028399077.5937638, 1028399077.5937638, 1028479722.7550542], [0.014090825, 0.01416563, 0.01416563, 0.014090825, 0.014090825]}, {[1026728042.2238628, 1026728042.2238628], [0.014144355, 0.014170555000000001]}, {[1060103621.4849387, 1060103621.4849387], [0.01421067, 0.01430368]}, {[928917483.6448978, 929054857.2098373], [0.014253335, 0.014292485]}, {[1020995471.866172, 1020995471.866172], [0.01425547, 0.014307074999999999]}, {[1050818739.1925838, 1050818739.1925838, 1050641119.2991557, 1050641119.2991557, 1050818739.1925838], [0.014321615, 0.014423374999999999, 0.014423374999999999, 0.014321615, 0.014321615]}, {[1060210906.3844512, 1060210906.3844512, 1060088056.261601, 1060088056.261601, 1060210906.3844512], [0.01437582, 0.014395664999999998, 0.014395664999999998, 0.01437582, 0.01437582]}, {[1010524208.2116058, 1010524208.2116058, 1010446688.8317609, 1010446688.8317609, 1010524208.2116058], [0.01440032, 0.014961515, 0.014961515, 0.01440032, 0.01440032]}, {[1067340749.8623314, 1067340749.8623314, 1067233912.2554936, 1067233912.2554936, 1067340749.8623314], [0.014432655, 0.014522705, 0.014522705, 0.014432655, 0.014432655]}, {[994154871.3947781, 994304336.1790955], [0.01444346, 0.014476125]}, {[996643673.8301789, 996643673.8301789, 996530423.5470532, 996530423.5470532, 996643673.8301789], [0.0144467, 0.01449745, 0.01449745, 0.0144467, 0.0144467]}, {[929162452.3956556, 929162452.3956556], [0.01447279, 0.014515215]}, {[984517369.6351253, 984599401.9622253], [0.01452572, 0.014625520000000001]}, {[1073152530.0637031, 1073152530.0637031], [0.014538525, 0.014646275]}, {[1082291065.6729505, 1082469758.1538203], [0.01461913, 0.014684885]}, {[989419092.0700991, 989419092.0700991, 989346496.7887924, 989346496.7887924, 989419092.0700991], [0.014661605, 0.01471253, 0.01471253, 0.014661605, 0.014661605]}, {[1054560346.3581073, 1054742969.627864], [0.01466516, 0.014765705]}, {[907652360.3992398, 907652360.3992398, 907562914.960957, 907562914.960957, 907652360.3992398], [0.014750235, 0.014900795, 0.014900795, 0.014750235, 0.014750235]}, {[1062189174.9203769, 1062189174.9203769], [0.01485058, 0.01492129]}, {[1026728042.2238628, 1026728042.2238628], [0.014901345, 0.014927545]}, {[927476484.2448008, 927613857.8097403], [0.015006225, 0.015045375]}, {[1021330874.2578875, 1021330874.2578875], [0.015073035, 0.01512464]}, {[1060251782.7954887, 1060251782.7954887, 1060128932.6726385, 1060128932.6726385, 1060251782.7954887], [0.01510531, 0.015125155, 0.015125155, 0.01510531, 0.01510531]}, {[992027316.0868192, 992176780.8711365], [0.01516978, 0.015202445]}, {[988830819.370068, 988830819.370068, 988758224.0887612, 988758224.0887612, 988830819.370068], [0.015357705, 0.01540863, 0.01540863, 0.015357705, 0.015357705]}, {[929162452.3956556, 929162452.3956556], [0.015363915, 0.015406340000000001]}, {[1082864717.4175386, 1082864717.4175386, 1082774950.8107162, 1082774950.8107162, 1082864717.4175386], [0.015532425, 0.01585597, 0.01585597, 0.015532425, 0.015532425]}, {[995507474.9163239, 995507474.9163239, 995394224.6331983, 995394224.6331983, 995507474.9163239], [0.015556975, 0.015607725000000001, 0.015607725000000001, 0.015556975, 0.015556975]}, {[1080469326.322043, 1080648018.8029127], [0.015607665, 0.01567342]}, {[1026728042.2238628, 1026728042.2238628], [0.01565833, 0.015684530000000002]}, {[928917483.6448978, 929054857.2098373], [0.01575912, 0.015798270000000003]}, {[984517369.6351253, 984599401.9622253], [0.01579842, 0.01589822]}, {[1073135024.1335804, 1073135024.1335804], [0.015822155, 0.015929905]}, {[1055565518.0981148, 1055748141.3678715], [0.015825595, 0.015926140000000002]}, {[1062189174.9203769, 1062189174.9203769], [0.015826695, 0.015897405000000003]}, {[1060210906.3844512, 1060210906.3844512, 1060088056.261601, 1060088056.261601, 1060210906.3844512], [0.0158348, 0.015854645, 0.015854645, 0.0158348, 0.0158348]}, {[1020995471.866172, 1020995471.866172], [0.015890605, 0.01594221]}, {[994154871.3947781, 994304336.1790955], [0.015896095, 0.01592876]}, {[1051290310.7105097, 1051290310.7105097, 1051112690.8170816, 1051112690.8170816, 1051290310.7105097], [0.01600832, 0.01611008, 0.01611008, 0.01600832, 0.01600832]}, {[989419092.0700991, 989419092.0700991, 989346496.7887924, 989346496.7887924, 989419092.0700991], [0.0160538, 0.016104725, 0.016104725, 0.0160538, 0.0160538]}, {[929162452.3956556, 929162452.3956556], [0.016255045, 0.016297469999999998]}, {[1067340749.8623314, 1067340749.8623314, 1067233912.2554936, 1067233912.2554936, 1067340749.8623314], [0.016371015, 0.016461065, 0.016461065, 0.016371015, 0.016371015]}, {[1026728042.2238628, 1026728042.2238628], [0.01641532, 0.01644152]}, {[927476484.2448008, 927613857.8097403], [0.01651201, 0.016551160000000002]}, {[1060251782.7954887, 1060251782.7954887, 1060128932.6726385, 1060128932.6726385, 1060251782.7954887], [0.01656429, 0.016584135, 0.016584135, 0.01656429, 0.01656429]}, {[1027479006.2384171, 1027479006.2384171, 1027398361.0771267, 1027398361.0771267, 1027479006.2384171], [0.016574735, 0.01664954, 0.01664954, 0.016574735, 0.016574735]}, {[1082291065.6729505, 1082469758.1538203], [0.016596205, 0.01666196]}, {[992027316.0868192, 992176780.8711365], [0.01662241, 0.016655075000000002]}, {[996643673.8301789, 996643673.8301789, 996530423.5470532, 996530423.5470532, 996643673.8301789], [0.01666725, 0.016718, 0.016718, 0.01666725, 0.01666725]}, {[1021330874.2578875, 1021330874.2578875], [0.01670817, 0.016759775]}, {[959254135.8898987, 959254135.8898987, 959109313.2975742, 959109313.2975742, 959254135.8898987], [0.01672565, 0.017115710000000003, 0.017115710000000003, 0.01672565, 0.01672565]}, {[988830819.370068, 988830819.370068, 988758224.0887612, 988758224.0887612, 988830819.370068], [0.0167499, 0.016800825000000002, 0.016800825000000002, 0.0167499, 0.0167499]}, {[1032360862.9064839, 1032360862.9064839, 1032279956.7576165, 1032279956.7576165, 1032360862.9064839], [0.01677671, 0.01724102, 0.01724102, 0.01677671, 0.01677671]}, {[1060103621.4849387, 1060103621.4849387], [0.016778205, 0.016871215000000002]}, {[1062189174.9203769, 1062189174.9203769], [0.016802805, 0.016873515000000002]}, {[909232485.1651794, 909232485.1651794, 909143039.7268966, 909143039.7268966, 909232485.1651794], [0.016957735, 0.017108295000000003, 0.017108295000000003, 0.016957735, 0.016957735]}, {[1054560346.3581073, 1054742969.627864], [0.016986025, 0.01708657]}, {[984517369.6351253, 984599401.9622253], [0.01707112, 0.01717092]}, {[1073152530.0637031, 1073152530.0637031], [0.01710579, 0.01721354]}, {[929162452.3956556, 929162452.3956556], [0.01714617, 0.017188594999999997]}, {[1026728042.2238628, 1026728042.2238628], [0.017172305, 0.017198505]}, {[928917483.6448978, 929054857.2098373], [0.0172649, 0.01730405]}, {[1060210906.3844512, 1060210906.3844512, 1060088056.261601, 1060088056.261601, 1060210906.3844512], [0.017293785, 0.01731363, 0.01731363, 0.017293785, 0.017293785]}, {[994154871.3947781, 994304336.1790955], [0.017348725, 0.01738139]}, {[989419092.0700991, 989419092.0700991, 989346496.7887924, 989346496.7887924, 989419092.0700991], [0.017446, 0.017496925, 0.017496925, 0.017446, 0.017446]}, {[1020995471.866172, 1020995471.866172], [0.017525735, 0.01757734]}, {[1080469326.322043, 1080648018.8029127], [0.017584745, 0.0176505]}, {[1050818739.1925838, 1050818739.1925838, 1050641119.2991557, 1050641119.2991557, 1050818739.1925838], [0.017695025, 0.017796785, 0.017796785, 0.017695025, 0.017695025]}, {[995507474.9163239, 995507474.9163239, 995394224.6331983, 995394224.6331983, 995507474.9163239], [0.017777525, 0.017828274999999998, 0.017828274999999998, 0.017777525, 0.017777525]}, {[1062189174.9203769, 1062189174.9203769], [0.01777892, 0.017849630000000002]}, {[1069922913.2514993, 1069922913.2514993, 1069753277.9673601, 1069753277.9673601, 1069922913.2514993], [0.01780574, 0.01812511, 0.01812511, 0.01780574, 0.01780574]}, {[1026728042.2238628, 1026728042.2238628], [0.017929295, 0.017955495000000002]}, {[927476484.2448008, 927613857.8097403], [0.01801779, 0.01805694]}, {[1060251782.7954887, 1060251782.7954887, 1060128932.6726385, 1060128932.6726385, 1060251782.7954887], [0.018023275, 0.01804312, 0.01804312, 0.018023275, 0.018023275]}, {[929162452.3956556, 929162452.3956556], [0.018037295, 0.018079719999999997]}, {[992027316.0868192, 992176780.8711365], [0.018075045, 0.018107710000000003]}, {[988830819.370068, 988830819.370068, 988758224.0887612, 988758224.0887612, 988830819.370068], [0.0181421, 0.018193025, 0.018193025, 0.0181421, 0.0181421]}, {[1055565518.0981148, 1055748141.3678715], [0.01814646, 0.018247005]}, {[1067340749.8623314, 1067340749.8623314, 1067233912.2554936, 1067233912.2554936, 1067340749.8623314], [0.01830937, 0.01839942, 0.01839942, 0.01830937, 0.01830937]}, {[1021330874.2578875, 1021330874.2578875], [0.0183433, 0.018394905]}, {[984517369.6351253, 984599401.9622253], [0.01834382, 0.01844362]}, {[1073135024.1335804, 1073135024.1335804], [0.01838942, 0.01849717]}, {[1082291065.6729505, 1082469758.1538203], [0.01857328, 0.018639035]}, {[1026728042.2238628, 1026728042.2238628], [0.018686285, 0.018712485]}, {[1060210906.3844512, 1060210906.3844512, 1060088056.261601, 1060088056.261601, 1060210906.3844512], [0.018752765, 0.018772610000000002, 0.018772610000000002, 0.018752765, 0.018752765]}, {[1062189174.9203769, 1062189174.9203769], [0.01875503, 0.01882574]}, {[928917483.6448978, 929054857.2098373], [0.01877068, 0.018809830000000003]}, {[994154871.3947781, 994304336.1790955], [0.01880136, 0.018834025]}, {[989419092.0700991, 989419092.0700991, 989346496.7887924, 989346496.7887924, 989419092.0700991], [0.0188382, 0.018889125, 0.018889125, 0.0188382, 0.0188382]}, {[996643673.8301789, 996643673.8301789, 996530423.5470532, 996530423.5470532, 996643673.8301789], [0.018887795, 0.018938544999999998, 0.018938544999999998, 0.018887795, 0.018887795]}, {[929162452.3956556, 929162452.3956556], [0.018928425, 0.018970849999999997]}, {[1028479722.7550542, 1028479722.7550542, 1028399077.5937638, 1028399077.5937638, 1028479722.7550542], [0.01905864, 0.019133445000000002, 0.019133445000000002, 0.01905864, 0.01905864]}, {[1083149040.2114863, 1083149040.2114863, 1083059273.6046643, 1083059273.6046643, 1083149040.2114863], [0.019133475, 0.019457020000000002, 0.019457020000000002, 0.019133475, 0.019133475]}, {[1020995471.866172, 1020995471.866172], [0.01916087, 0.019212475]}, {[907652360.3992398, 907652360.3992398, 907562914.960957, 907562914.960957, 907652360.3992398], [0.01916524, 0.0193158, 0.0193158, 0.01916524, 0.01916524]}, {[1054560346.3581073, 1054742969.627864], [0.01930689, 0.019407435]}, {[1060103621.4849387, 1060103621.4849387], [0.019345745, 0.019438755000000002]}, {[1051290310.7105097, 1051290310.7105097, 1051112690.8170816, 1051112690.8170816, 1051290310.7105097], [0.019381725, 0.019483485, 0.019483485, 0.019381725, 0.019381725]}, {[1026728042.2238628, 1026728042.2238628], [0.01944327, 0.01946947]}, {[1060251782.7954887, 1060251782.7954887, 1060128932.6726385, 1060128932.6726385, 1060251782.7954887], [0.019482255, 0.0195021, 0.0195021, 0.019482255, 0.019482255]}, {[927476484.2448008, 927613857.8097403], [0.019523575, 0.019562725000000003]}, {[992027316.0868192, 992176780.8711365], [0.019527675, 0.019560340000000002]}, {[988830819.370068, 988830819.370068, 988758224.0887612, 988758224.0887612, 988830819.370068], [0.019534295, 0.01958522, 0.01958522, 0.019534295, 0.019534295]}, {[1080469326.322043, 1080648018.8029127], [0.01956182, 0.019627575]}, {[984517369.6351253, 984599401.9622253], [0.01961652, 0.01971632]}, {[1073152530.0637031, 1073152530.0637031], [0.019673055, 0.019780805]}, {[1062189174.9203769, 1062189174.9203769], [0.019731145, 0.019801855]}, {[929162452.3956556, 929162452.3956556], [0.01981955, 0.019861974999999997]}, {[1021330874.2578875, 1021330874.2578875], [0.019978435, 0.02003004]}, {[995507474.9163239, 995507474.9163239, 995394224.6331983, 995394224.6331983, 995507474.9163239], [0.01999807, 0.02004882, 0.02004882, 0.01999807, 0.01999807]}, {[1026728042.2238628, 1026728042.2238628], [0.02020026, 0.02022646]}, {[1060210906.3844512, 1060210906.3844512, 1060088056.261601, 1060088056.261601, 1060210906.3844512], [0.02021175, 0.020231595, 0.020231595, 0.02021175, 0.02021175]}, {[989419092.0700991, 989419092.0700991, 989346496.7887924, 989346496.7887924, 989419092.0700991], [0.020230395, 0.020281320000000002, 0.020281320000000002, 0.020230395, 0.020230395]}, {[1067340749.8623314, 1067340749.8623314, 1067233912.2554936, 1067233912.2554936, 1067340749.8623314], [0.02024773, 0.02033778, 0.02033778, 0.02024773, 0.02024773]}, {[994154871.3947781, 994304336.1790955], [0.020253995, 0.02028666]}, {[928917483.6448978, 929054857.2098373], [0.020276465, 0.020315615000000002]}, {[1055565518.0981148, 1055748141.3678715], [0.020467325, 0.020567870000000002]}, {[1082291065.6729505, 1082469758.1538203], [0.020550355, 0.02061611]}, {[958900541.628188, 958900541.628188, 958736338.0157086, 958736338.0157086, 958900541.628188], [0.020635945, 0.021234085, 0.021234085, 0.020635945, 0.020635945]}, {[1062189174.9203769, 1062189174.9203769], [0.020707255, 0.020777965000000002]}, {[929162452.3956556, 929162452.3956556], [0.020710675, 0.0207531]}, {[1010524208.2116058, 1010524208.2116058, 1010446688.8317609, 1010446688.8317609, 1010524208.2116058], [0.020778575, 0.02133977, 0.02133977, 0.020778575, 0.020778575]}, {[1020995471.866172, 1020995471.866172], [0.020796, 0.020847604999999998]}, {[984517369.6351253, 984599401.9622253], [0.02088922, 0.02098902]}, {[988830819.370068, 988830819.370068, 988758224.0887612, 988758224.0887612, 988830819.370068], [0.020926495, 0.02097742, 0.02097742, 0.020926495, 0.020926495]}, {[1060251782.7954887, 1060251782.7954887, 1060128932.6726385, 1060128932.6726385, 1060251782.7954887], [0.02094124, 0.020961085, 0.020961085, 0.02094124, 0.02094124]}, {[1073135024.1335804, 1073135024.1335804], [0.020956685, 0.021064435]}, {[1026728042.2238628, 1026728042.2238628], [0.020957245, 0.020983445]}, {[992027316.0868192, 992176780.8711365], [0.02098031, 0.021012975]}, {[927476484.2448008, 927613857.8097403], [0.021029355, 0.021068505]}, {[1050818739.1925838, 1050818739.1925838, 1050641119.2991557, 1050641119.2991557, 1050818739.1925838], [0.02106843, 0.02117019, 0.02117019, 0.02106843, 0.02106843]}, {[996643673.8301789, 996643673.8301789, 996530423.5470532, 996530423.5470532, 996643673.8301789], [0.021108345, 0.021159095, 0.021159095, 0.021108345, 0.021108345]}, {[959254135.8898987, 959254135.8898987, 959109313.2975742, 959109313.2975742, 959254135.8898987], [0.02124135, 0.02163141, 0.02163141, 0.02124135, 0.02124135]}, {[909232485.1651794, 909232485.1651794, 909143039.7268966, 909143039.7268966, 909232485.1651794], [0.021372745, 0.021523305, 0.021523305, 0.021372745, 0.021372745]}, {[1080469326.322043, 1080648018.8029127], [0.021538895, 0.02160465]}, {[1027479006.2384171, 1027479006.2384171, 1027398361.0771267, 1027398361.0771267, 1027479006.2384171], [0.02154255, 0.021617355, 0.021617355, 0.02154255, 0.02154255]}, {[929162452.3956556, 929162452.3956556], [0.021601805, 0.02164423]}, {[1021330874.2578875, 1021330874.2578875], [0.021613565, 0.02166517]}, {[989419092.0700991, 989419092.0700991, 989346496.7887924, 989346496.7887924, 989419092.0700991], [0.021622595, 0.02167352, 0.02167352, 0.021622595, 0.021622595]}, {[1054560346.3581073, 1054742969.627864], [0.021627755, 0.0217283]}, {[1060210906.3844512, 1060210906.3844512, 1060088056.261601, 1060088056.261601, 1060210906.3844512], [0.02167073, 0.021690575, 0.021690575, 0.02167073, 0.02167073]}, {[1062189174.9203769, 1062189174.9203769], [0.02168337, 0.021754080000000002]}, {[994154871.3947781, 994304336.1790955], [0.021706625, 0.02173929]}, {[1026728042.2238628, 1026728042.2238628], [0.021714235, 0.021740435]}, {[928917483.6448978, 929054857.2098373], [0.021782245, 0.021821395]}, {[1060103621.4849387, 1060103621.4849387], [0.02191328, 0.02200629]}, {[1031645785.7104015, 1031645785.7104015, 1031564879.5615342, 1031564879.5615342, 1031645785.7104015], [0.021982915, 0.022447224999999998, 0.022447224999999998, 0.021982915, 0.021982915]}, {[984517369.6351253, 984599401.9622253], [0.02216192, 0.022261720000000002]}, {[1067340749.8623314, 1067340749.8623314, 1067233912.2554936, 1067233912.2554936, 1067340749.8623314], [0.02218609, 0.02227614, 0.02227614, 0.02218609, 0.02218609]}, {[995507474.9163239, 995507474.9163239, 995394224.6331983, 995394224.6331983, 995507474.9163239], [0.02221862, 0.02226937, 0.02226937, 0.02221862, 0.02221862]}, {[1073152530.0637031, 1073152530.0637031], [0.02224032, 0.02234807]}, {[988830819.370068, 988830819.370068, 988758224.0887612, 988758224.0887612, 988830819.370068], [0.022318695, 0.02236962, 0.02236962, 0.022318695, 0.022318695]}, {[1060251782.7954887, 1060251782.7954887, 1060128932.6726385, 1060128932.6726385, 1060251782.7954887], [0.02240022, 0.022420065, 0.022420065, 0.02240022, 0.02240022]}, {[1020995471.866172, 1020995471.866172], [0.022431135, 0.02248274]}, {[992027316.0868192, 992176780.8711365], [0.022432945, 0.02246561]}, {[1026728042.2238628, 1026728042.2238628], [0.02247122, 0.02249742]}, {[929162452.3956556, 929162452.3956556], [0.02249293, 0.022535355]}, {[1082291065.6729505, 1082469758.1538203], [0.022527435, 0.02259319]}, {[927476484.2448008, 927613857.8097403], [0.022535135, 0.022574285000000003]}, {[1062189174.9203769, 1062189174.9203769], [0.02265948, 0.02273019]}, {[1082864717.4175386, 1082864717.4175386, 1082774950.8107162, 1082774950.8107162, 1082864717.4175386], [0.02273453, 0.023058075, 0.023058075, 0.02273453, 0.02273453]}, {[1051290310.7105097, 1051290310.7105097, 1051112690.8170816, 1051112690.8170816, 1051290310.7105097], [0.022755135, 0.022856895, 0.022856895, 0.022755135, 0.022755135]}, {[1055565518.0981148, 1055748141.3678715], [0.022788185, 0.02288873]}, {[989419092.0700991, 989419092.0700991, 989346496.7887924, 989346496.7887924, 989419092.0700991], [0.02301479, 0.023065715, 0.023065715, 0.02301479, 0.02301479]}, {[1060210906.3844512, 1060210906.3844512, 1060088056.261601, 1060088056.261601, 1060210906.3844512], [0.023129715, 0.02314956, 0.02314956, 0.023129715, 0.023129715]}, {[994154871.3947781, 994304336.1790955], [0.02315926, 0.023191925000000002]}, {[1026728042.2238628, 1026728042.2238628], [0.02322821, 0.02325441]}, {[1021330874.2578875, 1021330874.2578875], [0.0232487, 0.023300305]}, {[928917483.6448978, 929054857.2098373], [0.02328803, 0.023327180000000003]}, {[996643673.8301789, 996643673.8301789, 996530423.5470532, 996530423.5470532, 996643673.8301789], [0.023328895, 0.023379644999999998, 0.023379644999999998, 0.023328895, 0.023328895]}, {[929162452.3956556, 929162452.3956556], [0.02338406, 0.023426485]}, {[984517369.6351253, 984599401.9622253], [0.02343462, 0.02353442]}, {[1080469326.322043, 1080648018.8029127], [0.02351597, 0.023581725]}, {[1073135024.1335804, 1073135024.1335804], [0.02352395, 0.0236317]}, {[907652360.3992398, 907652360.3992398, 907562914.960957, 907562914.960957, 907652360.3992398], [0.02358025, 0.02373081, 0.02373081, 0.02358025, 0.02358025]}, {[1062189174.9203769, 1062189174.9203769], [0.023635595, 0.023706305]}, {[988830819.370068, 988830819.370068, 988758224.0887612, 988758224.0887612, 988830819.370068], [0.02371089, 0.023761815, 0.023761815, 0.02371089, 0.02371089]}, {[1060251782.7954887, 1060251782.7954887, 1060128932.6726385, 1060128932.6726385, 1060251782.7954887], [0.023859205, 0.023879050000000002, 0.023879050000000002, 0.023859205, 0.023859205]}, {[992027316.0868192, 992176780.8711365], [0.023885575, 0.02391824]}, {[1054560346.3581073, 1054742969.627864], [0.02394862, 0.024049165]}, {[1026728042.2238628, 1026728042.2238628], [0.023985195, 0.024011395]}, {[1028479722.7550542, 1028479722.7550542, 1028399077.5937638, 1028399077.5937638, 1028479722.7550542], [0.02402646, 0.024101265, 0.024101265, 0.02402646, 0.02402646]}, {[927476484.2448008, 927613857.8097403], [0.02404092, 0.024080070000000002]}, {[1020995471.866172, 1020995471.866172], [0.024066265, 0.02411787]}, {[920932748.9465165, 920932748.9465165, 920784710.4565091, 920784710.4565091, 920932748.9465165], [0.02406716, 0.024682635, 0.024682635, 0.02406716, 0.02406716]}, {[1067340749.8623314, 1067340749.8623314, 1067233912.2554936, 1067233912.2554936, 1067340749.8623314], [0.024124445, 0.024214495000000003, 0.024214495000000003, 0.024124445, 0.024124445]}, {[929162452.3956556, 929162452.3956556], [0.024275185, 0.02431761]}, {[989419092.0700991, 989419092.0700991, 989346496.7887924, 989346496.7887924, 989419092.0700991], [0.02440699, 0.024457915, 0.024457915, 0.02440699, 0.02440699]}, {[995507474.9163239, 995507474.9163239, 995394224.6331983, 995394224.6331983, 995507474.9163239], [0.02443917, 0.02448992, 0.02448992, 0.02443917, 0.02443917]}, {[1050818739.1925838, 1050818739.1925838, 1050641119.2991557, 1050641119.2991557, 1050818739.1925838], [0.02444184, 0.0245436, 0.0245436, 0.02444184, 0.02444184]}, {[1060103621.4849387, 1060103621.4849387], [0.02448082, 0.02457383]}, {[1082291065.6729505, 1082469758.1538203], [0.02450451, 0.024570265]}, {[1060210906.3844512, 1060210906.3844512, 1060088056.261601, 1060088056.261601, 1060210906.3844512], [0.024588695, 0.02460854, 0.02460854, 0.024588695, 0.024588695]}, {[1062189174.9203769, 1062189174.9203769], [0.024611705, 0.024682415000000003]}, {[994154871.3947781, 994304336.1790955], [0.024611895, 0.024644560000000003]}, {[984517369.6351253, 984599401.9622253], [0.02470732, 0.024807120000000002]}, {[1026728042.2238628, 1026728042.2238628], [0.024742185, 0.024768385]}, {[928917483.6448978, 929054857.2098373], [0.02479381, 0.02483296]}, {[1073152530.0637031, 1073152530.0637031], [0.024807585, 0.024915335]}, {[1021330874.2578875, 1021330874.2578875], [0.02488383, 0.024935435]}, {[988830819.370068, 988830819.370068, 988758224.0887612, 988758224.0887612, 988830819.370068], [0.02510309, 0.025154015000000002, 0.025154015000000002, 0.02510309, 0.02510309]}, {[1055565518.0981148, 1055748141.3678715], [0.02510905, 0.025209595]}, {[929162452.3956556, 929162452.3956556], [0.02516631, 0.025208735]}, {[1060251782.7954887, 1060251782.7954887, 1060128932.6726385, 1060128932.6726385, 1060251782.7954887], [0.025318185, 0.02533803, 0.02533803, 0.025318185, 0.025318185]}, {[992027316.0868192, 992176780.8711365], [0.02533821, 0.025370875]}, {[1080469326.322043, 1080648018.8029127], [0.02549305, 0.025558805]}, {[1026728042.2238628, 1026728042.2238628], [0.025499175, 0.025525375]}, {[927476484.2448008, 927613857.8097403], [0.0255467, 0.02558585]}, {[996643673.8301789, 996643673.8301789, 996530423.5470532, 996530423.5470532, 996643673.8301789], [0.02554944, 0.02560019, 0.02560019, 0.02554944, 0.02554944]}, {[1062189174.9203769, 1062189174.9203769], [0.02558782, 0.025658530000000002]}, {[1020995471.866172, 1020995471.866172], [0.0257014, 0.025753005]}, {[959254135.8898987, 959254135.8898987, 959109313.2975742, 959109313.2975742, 959254135.8898987], [0.02575705, 0.02614711, 0.02614711, 0.02575705, 0.02575705]}, {[909232485.1651794, 909232485.1651794, 909143039.7268966, 909143039.7268966, 909232485.1651794], [0.025787755, 0.025938315, 0.025938315, 0.025787755, 0.025787755]}, {[989419092.0700991, 989419092.0700991, 989346496.7887924, 989346496.7887924, 989419092.0700991], [0.025799185, 0.02585011, 0.02585011, 0.025799185, 0.025799185]}, {[984517369.6351253, 984599401.9622253], [0.02598002, 0.02607982]}, {[1060210906.3844512, 1060210906.3844512, 1060088056.261601, 1060088056.261601, 1060210906.3844512], [0.02604768, 0.026067525, 0.026067525, 0.02604768, 0.02604768]}, {[929162452.3956556, 929162452.3956556], [0.02605744, 0.026099865]}, {[1067340749.8623314, 1067340749.8623314, 1067233912.2554936, 1067233912.2554936, 1067340749.8623314], [0.026062805, 0.026152855000000003, 0.026152855000000003, 0.026062805, 0.026062805]}, {[994154871.3947781, 994304336.1790955], [0.026064525, 0.026097190000000003]}, {[1073135024.1335804, 1073135024.1335804], [0.02609122, 0.02619897]}, {[1051290310.7105097, 1051290310.7105097, 1051112690.8170816, 1051112690.8170816, 1051290310.7105097], [0.026128545, 0.026230305, 0.026230305, 0.026128545, 0.026128545]}, {[1026728042.2238628, 1026728042.2238628], [0.02625616, 0.02628236]}, {[1054560346.3581073, 1054742969.627864], [0.026269485, 0.02637003]}, {[928917483.6448978, 929054857.2098373], [0.02629959, 0.026338740000000003]}, {[1083149040.2114863, 1083149040.2114863, 1083059273.6046643, 1083059273.6046643, 1083149040.2114863], [0.02633558, 0.026659125000000002, 0.026659125000000002, 0.02633558, 0.02633558]}, {[1082291065.6729505, 1082469758.1538203], [0.026481585, 0.02654734]}, {[988830819.370068, 988830819.370068, 988758224.0887612, 988758224.0887612, 988830819.370068], [0.026495285, 0.02654621, 0.02654621, 0.026495285, 0.026495285]}, {[1027479006.2384171, 1027479006.2384171, 1027398361.0771267, 1027398361.0771267, 1027479006.2384171], [0.02651037, 0.026585175, 0.026585175, 0.02651037, 0.02651037]}, {[1021330874.2578875, 1021330874.2578875], [0.026518965, 0.026570569999999998]}, {[1062189174.9203769, 1062189174.9203769], [0.02656393, 0.02663464]}, {[995507474.9163239, 995507474.9163239, 995394224.6331983, 995394224.6331983, 995507474.9163239], [0.026659715, 0.026710465, 0.026710465, 0.026659715, 0.026659715]}, {[1071939451.6053249, 1071939451.6053249, 1071769816.3211857, 1071769816.3211857, 1071939451.6053249], [0.026720695, 0.027040065, 0.027040065, 0.026720695, 0.026720695]}, {[1060251782.7954887, 1060251782.7954887, 1060128932.6726385, 1060128932.6726385, 1060251782.7954887], [0.02677717, 0.026797015, 0.026797015, 0.02677717, 0.02677717]}, {[992027316.0868192, 992176780.8711365], [0.026790845, 0.026823510000000002]}, {[929162452.3956556, 929162452.3956556], [0.026948565, 0.02699099]}, {[1026728042.2238628, 1026728042.2238628], [0.02701315, 0.02703935]}, {[1060103621.4849387, 1060103621.4849387], [0.027048355, 0.027141365]}, {[927476484.2448008, 927613857.8097403], [0.02705248, 0.027091630000000002]}, {[1010524208.2116058, 1010524208.2116058, 1010446688.8317609, 1010446688.8317609, 1010524208.2116058], [0.02715683, 0.027718025, 0.027718025, 0.02715683, 0.02715683]}, {[1032360862.9064839, 1032360862.9064839, 1032279956.7576165, 1032279956.7576165, 1032360862.9064839], [0.02718912, 0.02765343, 0.02765343, 0.02718912, 0.02718912]}, {[989419092.0700991, 989419092.0700991, 989346496.7887924, 989346496.7887924, 989419092.0700991], [0.027191385, 0.02724231, 0.02724231, 0.027191385, 0.027191385]}, {[984517369.6351253, 984599401.9622253], [0.02725272, 0.02735252]}, {[1020995471.866172, 1020995471.866172], [0.02733653, 0.027388135]}, {[1073152530.0637031, 1073152530.0637031], [0.02737485, 0.0274826]}, {[1055565518.0981148, 1055748141.3678715], [0.027429915, 0.02753046]}, {[1080469326.322043, 1080648018.8029127], [0.027470125, 0.027535880000000002]}, {[1060210906.3844512, 1060210906.3844512, 1060088056.261601, 1060088056.261601, 1060210906.3844512], [0.02750666, 0.027526505, 0.027526505, 0.02750666, 0.02750666]}, {[994154871.3947781, 994304336.1790955], [0.02751716, 0.027549825]}, {[1062189174.9203769, 1062189174.9203769], [0.027540045, 0.027610755]}, {[996643673.8301789, 996643673.8301789, 996530423.5470532, 996530423.5470532, 996643673.8301789], [0.02776999, 0.02782074, 0.02782074, 0.02776999, 0.02776999]}]
  in  "run it again when done":bool=TRUE
  in  "run 2":bool
  out "dds free":bool[][](array[boolean])=[[TRUE, TRUE, TRUE, FALSE, TRUE, TRUE, TRUE, TRUE, TRUE, TRUE, TRUE, TRUE, TRUE, TRUE, TRUE, TRUE], [TRUE, TRUE, TRUE, FALSE, TRUE, TRUE, TRUE, TRUE, TRUE, TRUE, TRUE, TRUE, TRUE, TRUE, TRUE, TRUE], [TRUE, FALSE, TRUE, TRUE, TRUE, TRUE, TRUE, TRUE, TRUE, TRUE, TRUE, TRUE, TRUE, TRUE, TRUE, TRUE], [TRUE, FALSE, TRUE, TRUE, TRUE, TRUE, TRUE, TRUE, TRUE, TRUE, TRUE, TRUE, TRUE, TRUE, TRUE, TRUE], [FALSE, TRUE, TRUE, TRUE, TRUE, TRUE, TRUE, TRUE, TRUE, TRUE, TRUE, TRUE, TRUE, TRUE, TRUE, TRUE], [TRUE, TRUE, TRUE, TRUE, TRUE, TRUE, TRUE, TRUE, TRUE, TRUE, TRUE, TRUE, TRUE, TRUE, TRUE, TRUE]]
  out "pulse transmitted":u32[](array[numeric])=[252201, 252201, 252201, 252202, 252202, 0]
  out "clocks":dbl[](array[numeric])=[13.97066897, 13.97068317, 13.970729385, 13.970738995, 13.97078035, 13.970789675]
  out "lost sampels":u32
  # "available modulations:"
  # "csv coloms:\nt_start(sec)\nf_Hz\nduration (sec)\namp(dB)\nmod type\nmod_depth (Hz)\ndiraction (deg)"
  # "mod type"
  # "setup:\npxi with 5785 cards"
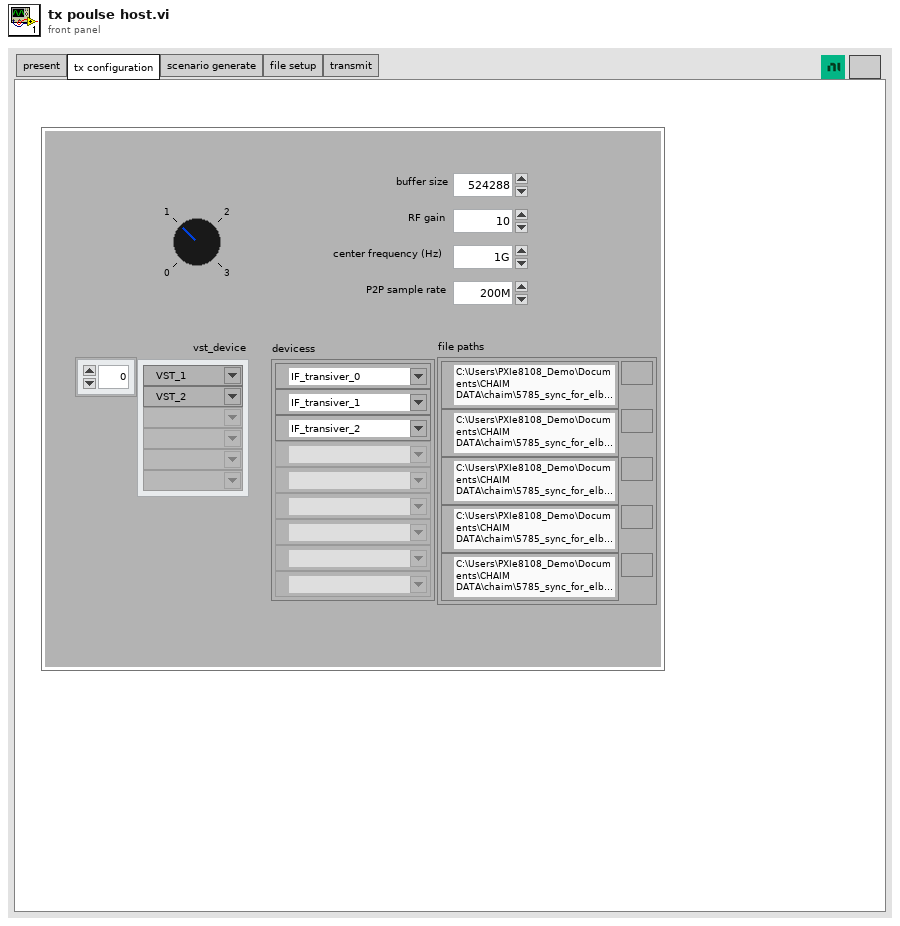
[diagram p1: front panel]
types:
  T1 = enum32{"present", "tx configuration", "scenario generate", "file setup", "transmit"}
  T2 = typedef "nirio_resource_hc.ctl" = tag
  T3 = cluster{"vst_device":refnum<k15>[], "file paths":path[], "RF gain ":dbl, "devicess ":T2[], "buffer size":u32, "center frequency (Hz) ":dbl, "Dial":u8, "P2P sample rate":dbl}
  T4 = enum32{"emitters parameters", "user manually created emitters", "CSV to TDMS"}
  T5 = typedef "random_limits.ctl" = cluster{"DOA range ":cluster{dbl, dbl}, "modulation depth":cluster{dbl, dbl}, "num of hoopers":i32, "num of frequncyes":cluster{i32, i32}, "QPSK":bool, "BPSK":bool, "LFM":bool, "CW":bool, "     f band range":cluster{dbl, dbl}, "D.C range":cluster{dbl, dbl}, "hop rate range":cluster{dbl, dbl}, "span range ":cluster{dbl, dbl}, "amp range":cluster{dbl, dbl}, "start time (sec)":dbl, "end time (sec)":dbl}
  T6 = typedef "emitter params.ctl" = cluster{"f set":dbl[], "hop rate (Hz)":dbl, "d.c.":dbl, "amp (dB)":dbl, "mod type":T7, "mod depth":dbl, "DOA":dbl, "t start":dbl, "t end":dbl}
  T7 = typedef "mode_type.ctl" = enum8{"CW", "NC - CW", "NC - cw", "LFM", "BPSK", "QPSK"}
  T8 = cluster{"PSK Color":u32, "LFM Color":u32, "CW Color":u32}
  T9 = typedef "secnario config.ctl" = cluster{"devicess 2":T2[], "file paths":path[], "buffer size":u32, "Fs  FPGA":dbl, "SPC":dbl, "center frequency (Hz) ":dbl, "t clock ref":refnum<k20>[], "fpga rfe":refnum<k20>[], "tdms refs":refnum<k34>[], "niUsrpRio Session (out)":T10, "RF gain ":i32, "mode":u8, "vst_device":refnum<k15>[], "IQ_rare_p2p":dbl, "stream sesion P2P":refnum<k20>[]}
  T10 = typedef "niUsrpRio Config v1 Host.lvlib/niUsrpRio Session.ctl" = cluster{"FPGA Interface":refnum<k20>, "RIO Interface Number":u32, "Data Clock Rate":u32, "FPGA Data Clock Rate":u32, "Global Settings Register Bus":T11, "Radio 0 Settings Register Bus":T11, "Radio 1 Settings Register Bus":T11, "Radio Settings Bus Semaphore":T12, "DB Queues":T13[], "Characterization Data Valid?":bool, "EEPROM Header":T14, "Device Data Header":T15, "EEPROM Characterization Header":T16, "Characterization Data":T17[], "FPGA Current Version":u32, "FPGA Oldest Compatible Version":u32, "Fixed Logic Current Version":u32, "Fixed Logic Oldest Compatible Version":u32, "FPGA Radio Settings Bus Current Version":u32, "FPGA Radio Settings Bus Oldest Compatible Version":u32, "FPGA Board Config Current Version":u32, "FPGA Board Config Oldest Compatible Version":u32, "Daughterboard Clock Rate":u32, "daughterboard configuration session handles":u64[]}
  T11 = typedef "niInstr Register Bus v0 Host.lvlib/Register Bus Session.ctl" = refnum<queue>
  T12 = typedef "Semaphore RefNum" = refnum<k1>
  T13 = typedef "niUsrpRio Config v1 Host.lvlib/DB Queue Reference.ctl" = refnum<queue>
  T14 = typedef "niUsrpRio Config v1 Host.lvlib/EEPROM Header.ctl" = cluster{"Checksum":u32, "Product Code":u16, "Hardware Current Version":u16, "Hardware Oldest Compatible Version":u16, "EEPROM Map Current Version":u16, "EEPROM Map Oldest Compatible Version":u16, "User Password":string, "Pointer to Factory Header":u32, "Pointer to User Header":u32, "Recommended Interval":u16, "Number of Reserved Bytes":i32, "Number of Daughterboards":u8, "Daughterboard IDs":u16[], "Daughterboard Serial Numbers":string[]}
  T15 = typedef "niUsrpRio Config v1 Host.lvlib/EEPROM Device Data Header.ctl" = cluster{"Checksum":u32, "Number of Channels":u8, "Number of Gain Settings":u16[], "Pointer to Characterization Data":u32[], "Number of Reserved Bytes":i32, "Number of Frequencies":u16[]}
  T16 = typedef "niUsrpRio Config v1 Host.lvlib/EEPROM Characterization Header.ctl" = cluster{"Checksum":u32, "Date":timestamp, "Temperature":sgl, "Misc. Info":string, "Pointer to Device Data Header":u32, "Number of Reserved Bytes":i32}
  T17 = typedef "niUsrpRio Config v1 Host.lvlib/Characterization Data.ctl" = cluster{"Gains[dB]":dbl[], "Frequencies [Hz]":dbl[], "IQ Imbalance Table":T18[], "Measured Gains[dB]":dbl[][]}
  T18 = typedef "niUsrpRio Config v1 Host.lvlib/IQ Imbalance.ctl" = cluster{"Gain Imbalance [linear]":dbl, "Phase Imbalance [radians]":dbl, "Offset":cdb}
  T19 = typedef "pdw.ctl" = cluster{"PW":u32, "frequency shift":fxp<+/-,48,0>, "amp":fxp<+/-,18,1>, "mode type":T7, "mode depth":u32, "mode filter":u8, "phase shift":fxp<+/-,16,1>, "pulse shape filter":u8}
  T20 = typedef "PDW_lv2.ctl" = cluster{"t start":dbl, "frequency (Hz)":dbl, "duration (sec)":dbl, "amp (lin)":dbl, "mod type":T7, "mod depth":dbl, "phase (rad)":dbl[]}
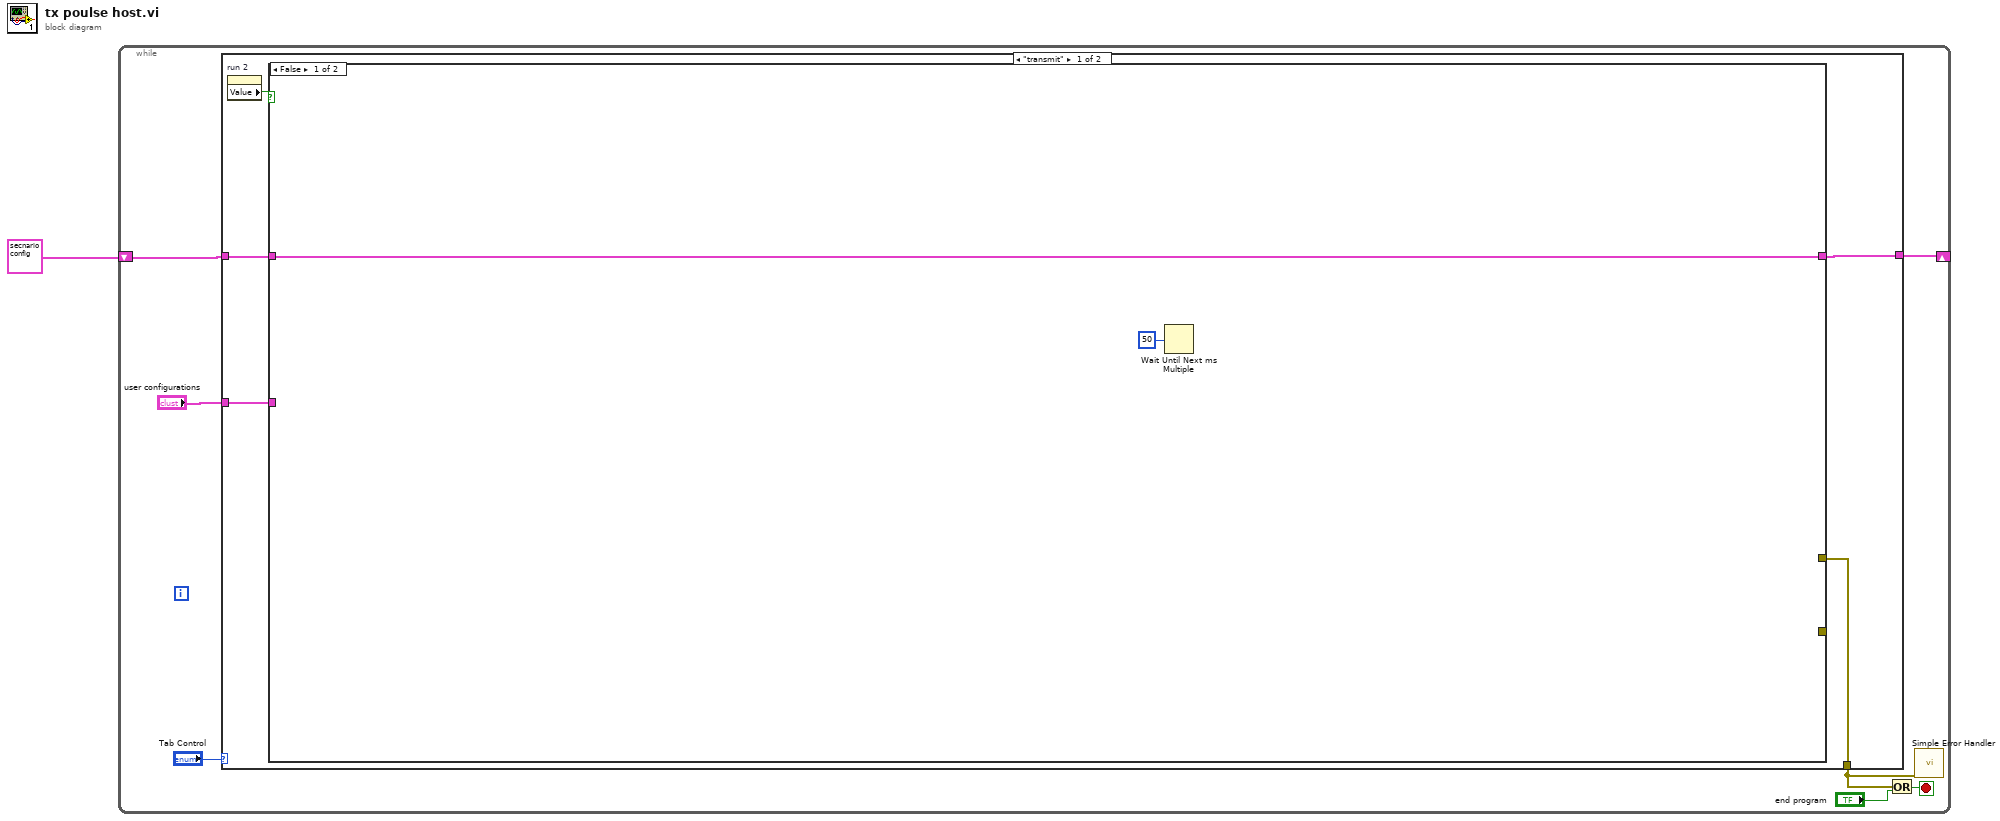
[diagram p0: block diagram]
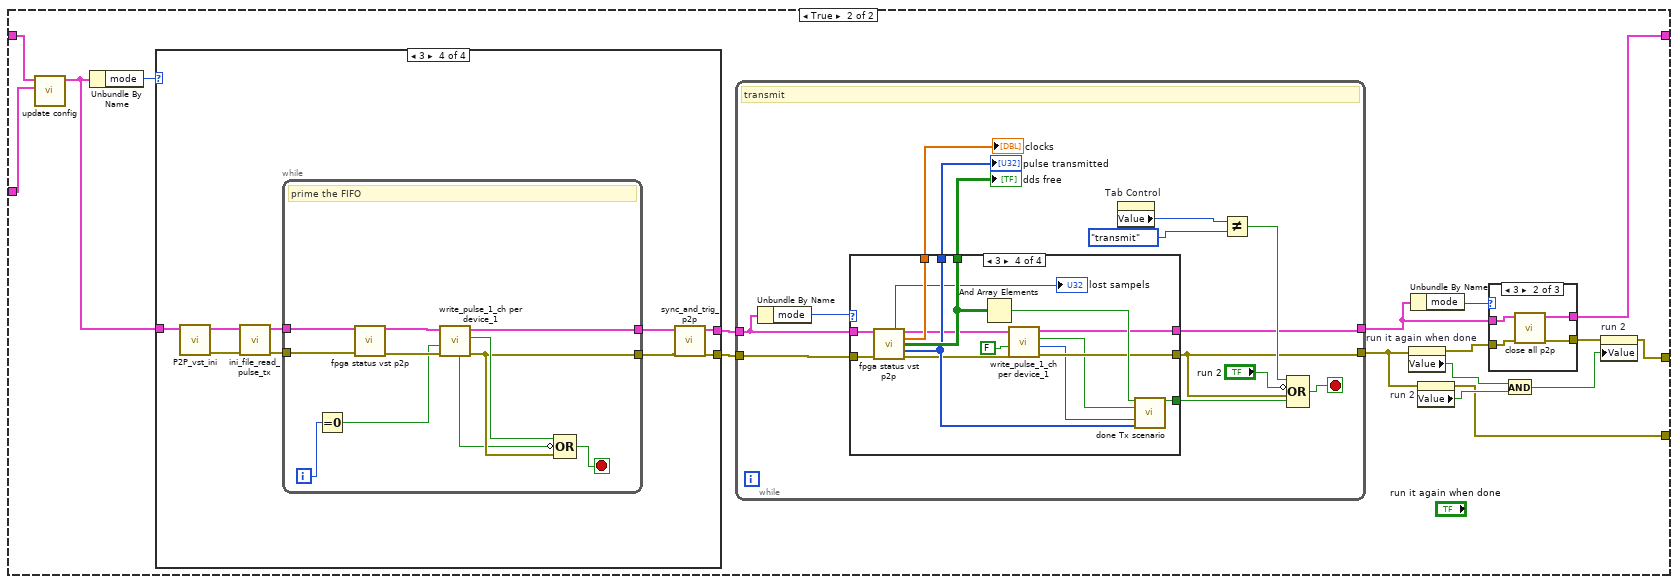
[diagram p2: hidden frame]
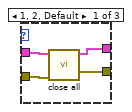
[diagram p3: hidden frame]
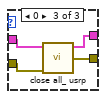
[diagram p4: hidden frame]
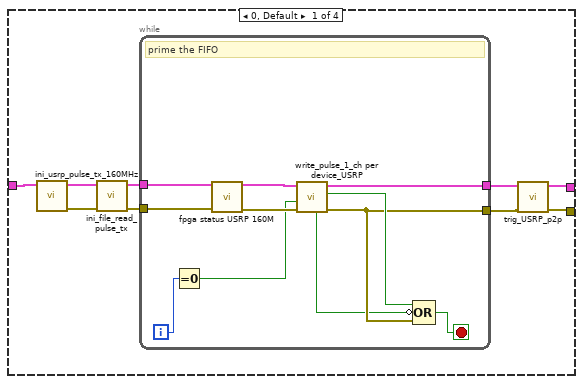
[diagram p5: hidden frame]
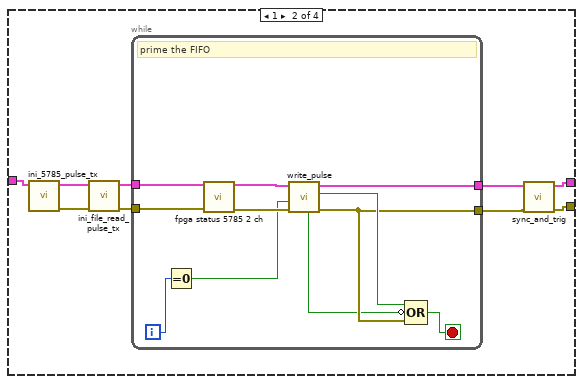
[diagram p6: hidden frame]
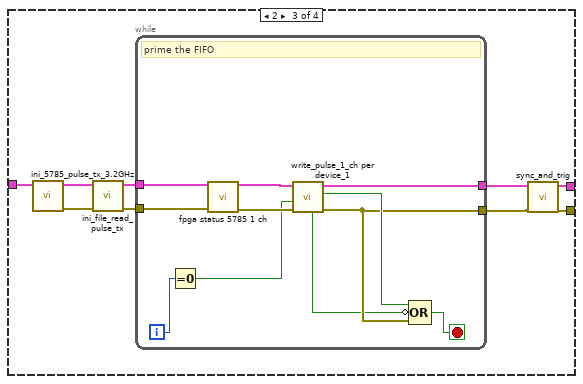
[diagram p7: hidden frame]
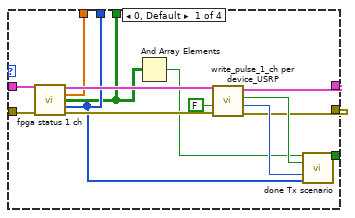
[diagram p8: hidden frame]
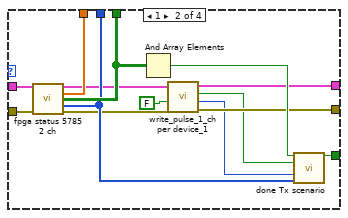
[diagram p9: hidden frame]
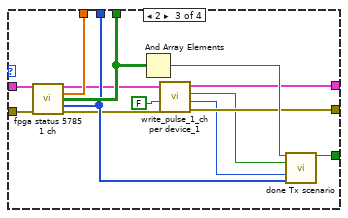
[diagram p10: hidden frame]
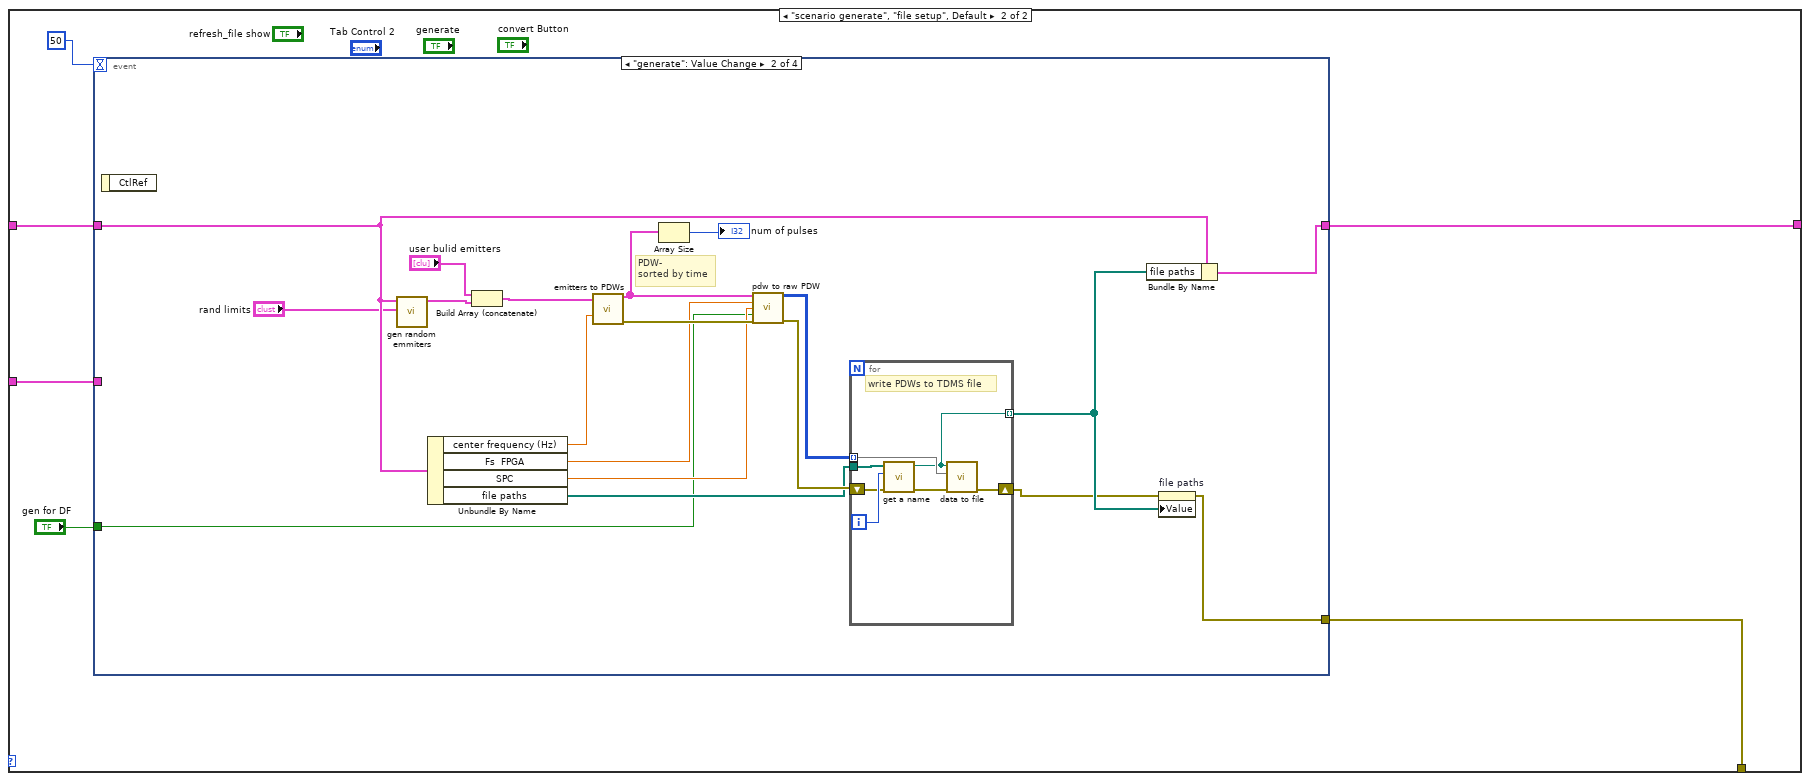
[diagram p11: hidden frame]
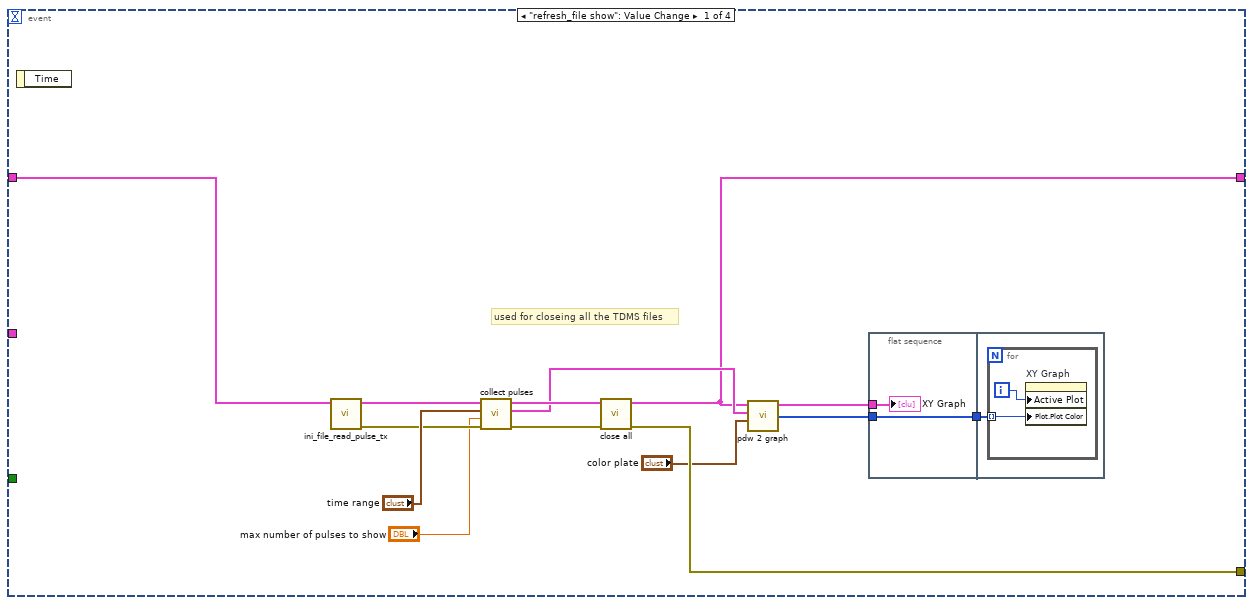
[diagram p12: hidden frame]
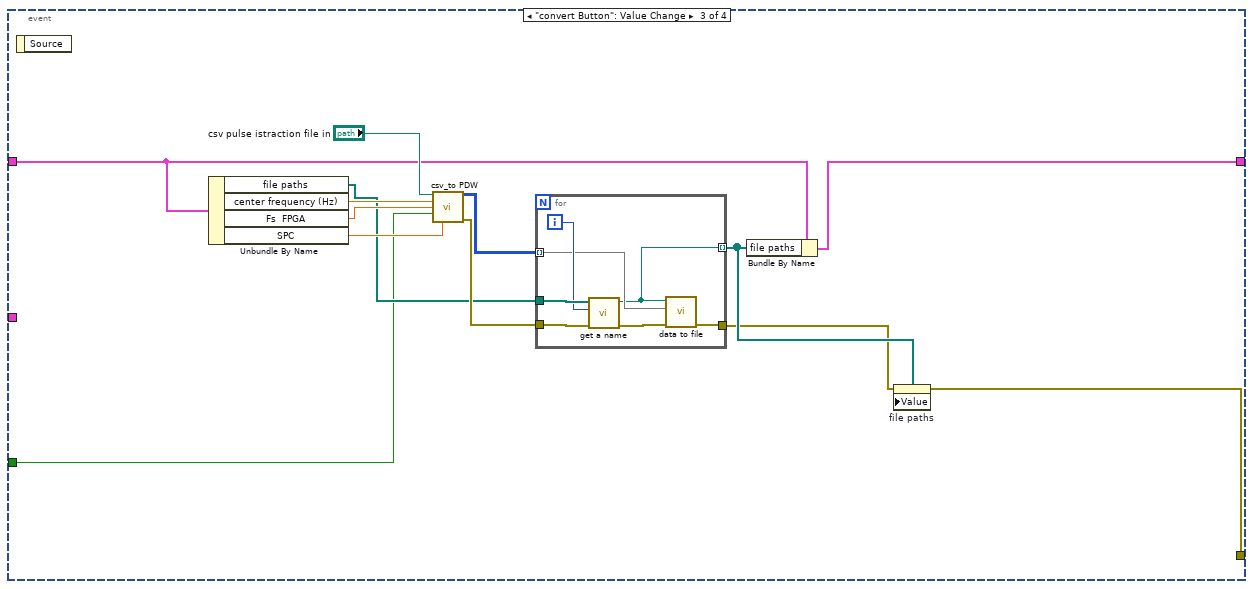
[diagram p13: hidden frame]
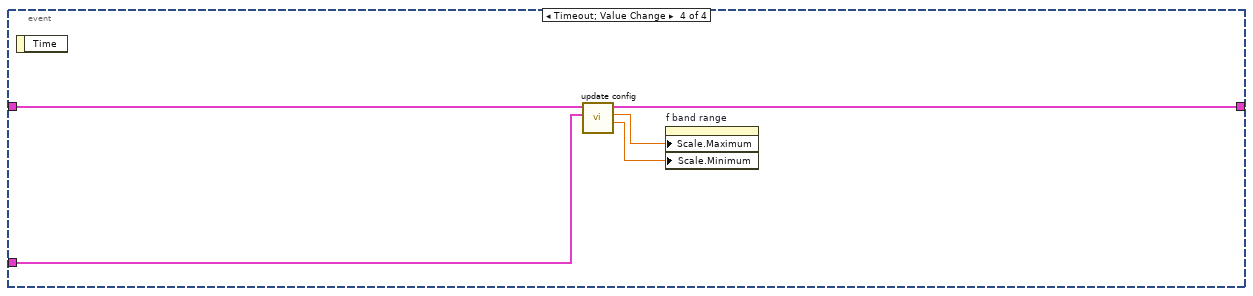
[diagram p14: hidden frame]
diagram:
  n1 = while {
    shift-right: [w5] -> _
    shift-left: T9 {"devicess 2"=["IF_transiver_1", "IF_transiver_2"], "file paths"=[path "C:/Users/PXIe8108_Demo/Documents/CHAIM DATA/chaim/5785_sync_for_elbit/data/pdw_test_file.tdms", path "C:/Users/PXIe8108_Demo/Documents/CHAIM DATA/chaim/5785_sync_for_elbit/data/pdw_test_file.tdms", path "C:/Users/PXIe8108_Demo/Documents/CHAIM DATA/chaim/5785_sync_for_elbit/data/pdw_test_file.tdms", path "C:/Users/PXIe8108_Demo/Documents/CHAIM DATA/chaim/5785_sync_for_elbit/data/pdw_test_file.tdms"], "buffer size"=524288, "Fs  FPGA"=200000000.0, "SPC"=1.0, "center frequency (Hz) "=1000000000.0, "t clock ref"=[], "fpga rfe"=[], "tdms refs"=[], "niUsrpRio Session (out)"={"FPGA Interface"=refnum, "RIO Interface Number"=0, "Data Clock Rate"=0, "FPGA Data Clock Rate"=0, "Global Settings Register Bus"=refnum, "Radio 0 Settings Register Bus"=refnum, "Radio 1 Settings Register Bus"=refnum, "Radio Settings Bus Semaphore"=refnum, "DB Queues"=[], "Characterization Data Valid?"=FALSE, "EEPROM Header"={"Checksum"=0, "Product Code"=0, "Hardware Current Version"=0, "Hardware Oldest Compatible Version"=0, "EEPROM Map Current Version"=0, "EEPROM Map Oldest Compatible Version"=0, "User Password"="", "Pointer to Factory Header"=0, "Pointer to User Header"=0, "Recommended Interval"=0, "Number of Reserved Bytes"=9, "Number of Daughterboards"=0, "Daughterboard IDs"=[], "Daughterboard Serial Numbers"=[]}, "Device Data Header"={"Checksum"=0, "Number of Channels"=0, "Number of Gain Settings"=[], "Pointer to Characterization Data"=[], "Number of Reserved Bytes"=27, "Number of Frequencies"=[]}, "EEPROM Characterization Header"={"Checksum"=0, "Date"=timestamp(0 s since 1904-01-01), "Temperature"=0.0, "Misc. Info"="", "Pointer to Device Data Header"=0, "Number of Reserved Bytes"=28}, "Characterization Data"=[], "FPGA Current Version"=0, "FPGA Oldest Compatible Version"=0, "Fixed Logic Current Version"=0, "Fixed Logic Oldest Compatible Version"=0, "FPGA Radio Settings Bus Current Version"=0, "FPGA Radio Settings Bus Oldest Compatible Version"=0, "FPGA Board Config Current Version"=0, "FPGA Board Config Oldest Compatible Version"=0, "Daughterboard Clock Rate"=0, "daughterboard configuration session handles"=[]}, "RF gain "=10, "mode"=2, "vst_device"=[], "IQ_rare_p2p"=200000000.0, "stream sesion P2P"=[]} ("secnario config") -> [w6]
    stop <- w7 stop-if-true
    n2 = case shown="\"transmit\"" "Tab Control" {
      tunnel: [w12 w200] -> w2
      tunnel: w6 -> [w11 w198]
      tunnel: [w10 w199] -> w5
      tunnel: "user configurations" -> [w9 w197]
      frame "transmit" {
        n3 = property on="run 2" class="Bool (strict)"() -> ("Value"=w13:bool)  [unwired: 2 in, 2 out]
        n4 = case shown="False" w13 {
          tunnel: [_ w31] -> w12
          tunnel: w11 -> [w14 w18]
          tunnel: [w14 w19] -> w10
          tunnel: [_ w20] -> _
          tunnel: w9 -> [_ w16]
          frame False {
            n5 = Wait Until Next ms Multiple(millisecond multiple=u32 50) -> ()  [unwired: 1 out]
          }
          frame True {
            n6 = call "update config.vi"("user configurations"=w16, "secnario config in"=w18) -> ("secnario config out"=w17:T9)  [unwired: 7 in, 2 out]
            n7 = Unbundle By Name(w17) -> ("mode"=w28:u8)
            n8 = case shown="3" w28 {
              tunnel: w17 -> [w47 w72 w87 w107]
              tunnel: [w46 w66 w86 w106] -> w30
              tunnel: [w45 w65 w85 w105] -> w29
              frame 0, Default {
                n9 = call "ini_usrp_pulse_tx_160MHz.vi"("secnario config"=w47) -> ("error out"=w53:errorcluster, "secnario config"=w52:T9)  [unwired: 9 in]
                n10 = call "ini_file_read_pulse_tx.vi"("error in (no error)"=w53, "secnario config"=w52) -> ("error out"=w50:errorcluster, "output cluster"=w51:T9)  [unwired: 8 in]
                n11 = while {
                  tunnel: w51 -> [w64]
                  tunnel: w50 -> [w63]
                  tunnel: [w59] -> w49
                  tunnel: [w56] -> w48
                  i -> [w62]
                  stop <- w55 stop-if-true
                  # "prime the FIFO"
                  n12 = Equal To 0?(x=w62) -> (x = 0?=w58:bool)
                  n13 = call "fpga status USRP 160M.vi"("secnario config"=w64, "error in (no error)"=w63) -> ("secnario config"=w61:T9, "error out"=w60:errorcluster)  [unwired: 9 in, 3 out]
                  n14 = call "write_pulse_1_ch per device_USRP.vi"("error in"=w60, "first call"=w58, "secnario config"=w61) -> ("error out"=w56:errorcluster, "done write files"=w57:bool, "output cluster"=w59:T9, "room on the FIFO"=w54:bool)  [unwired: 4 in, 1 out]
                  n15 = Compound Arithmetic op=OR(w57, invert w54, w56) -> (w55:bool)
                }
                n16 = call "trig_USRP_p2p.vi"("error in (no error)"=w48, "secnario config"=w49) -> ("error out"=w45:errorcluster, "secnario config 2"=w46:T9)  [unwired: 8 in]
              }
              frame 1 {
                n17 = call "ini_5785_pulse_tx.vi"("secnario config 2"=w72) -> ("error out"=w73:errorcluster, "secnario config"=w71:T9)  [unwired: 9 in]
                n18 = call "ini_file_read_pulse_tx.vi"("error in (no error)"=w73, "secnario config"=w71) -> ("error out"=w69:errorcluster, "output cluster"=w70:T9)  [unwired: 8 in]
                n19 = while {
                  tunnel: w70 -> [w84]
                  tunnel: w69 -> [w83]
                  tunnel: [w79] -> w68
                  tunnel: [w76] -> w67
                  i -> [w82]
                  stop <- w75 stop-if-true
                  # "prime the FIFO"
                  n20 = Equal To 0?(x=w82) -> (x = 0?=w78:bool)
                  n21 = call "fpga status 5785 2 ch.vi"("secnario config"=w84, "error in (no error)"=w83) -> ("secnario config"=w81:T9, "error out"=w80:errorcluster)  [unwired: 9 in, 3 out]
                  n22 = call "write_pulse.vi"("error in"=w80, "first call"=w78, "secnario config"=w81) -> ("error out"=w76:errorcluster, "done write files"=w77:bool, "output cluster"=w79:T9, "room on the FIFO"=w74:bool)  [unwired: 4 in, 1 out]
                  n23 = Compound Arithmetic op=OR(w77, invert w74, w76) -> (w75:bool)
                }
                n24 = call "sync_and_trig.vi"("error in (no error)"=w67, "secnario config"=w68) -> ("error out"=w65:errorcluster, "secnario config 2"=w66:T9)  [unwired: 8 in]
              }
              frame 2 {
                n25 = call "ini_5785_pulse_tx_3.2GHz.vi"("secnario config"=w87) -> ("error out"=w93:errorcluster, "secnario config"=w92:T9)  [unwired: 9 in]
                n26 = call "ini_file_read_pulse_tx.vi"("error in (no error)"=w93, "secnario config"=w92) -> ("error out"=w90:errorcluster, "output cluster"=w91:T9)  [unwired: 8 in]
                n27 = while {
                  tunnel: w91 -> [w104]
                  tunnel: w90 -> [w103]
                  tunnel: [w99] -> w89
                  tunnel: [w96] -> w88
                  i -> [w102]
                  stop <- w95 stop-if-true
                  # "prime the FIFO"
                  n28 = Equal To 0?(x=w102) -> (x = 0?=w98:bool)
                  n29 = call "fpga status 5785 1 ch.vi"("secnario config"=w104, "error in (no error)"=w103) -> ("secnario config"=w101:T9, "error out"=w100:errorcluster)  [unwired: 9 in, 3 out]
                  n30 = call "write_pulse_1_ch per device_1.vi"("error in"=w100, "first call"=w98, "secnario config"=w101) -> ("error out"=w96:errorcluster, "done write files"=w97:bool, "output cluster"=w99:T9, "room on the FIFO"=w94:bool)  [unwired: 4 in, 1 out]
                  n31 = Compound Arithmetic op=OR(w97, invert w94, w96) -> (w95:bool)
                }
                n32 = call "sync_and_trig.vi"("error in (no error)"=w88, "secnario config"=w89) -> ("error out"=w85:errorcluster, "secnario config 2"=w86:T9)  [unwired: 8 in]
              }
              frame 3 {
                n33 = call "P2P_vst_ini.vi"("secnario config"=w107) -> ("error out"=w113:errorcluster, "secnario config"=w112:T9)  [unwired: 9 in]
                n34 = call "ini_file_read_pulse_tx.vi"("error in (no error)"=w113, "secnario config"=w112) -> ("error out"=w110:errorcluster, "output cluster"=w111:T9)  [unwired: 8 in]
                n35 = while {
                  tunnel: w111 -> [w124]
                  tunnel: w110 -> [w123]
                  tunnel: [w119] -> w109
                  tunnel: [w116] -> w108
                  i -> [w122]
                  stop <- w115 stop-if-true
                  # "prime the FIFO"
                  n36 = Equal To 0?(x=w122) -> (x = 0?=w118:bool)
                  n37 = call "fpga status vst p2p.vi"("secnario config"=w124, "error in (no error)"=w123) -> ("secnario config"=w121:T9, "error out"=w120:errorcluster)  [unwired: 8 in, 4 out]
                  n38 = call "write_pulse_1_ch per device_1.vi"("error in"=w120, "first call"=w118, "secnario config"=w121) -> ("error out"=w116:errorcluster, "done write files"=w117:bool, "output cluster"=w119:T9, "room on the FIFO"=w114:bool)  [unwired: 4 in, 1 out]
                  n39 = Compound Arithmetic op=OR(w117, invert w114, w116) -> (w115:bool)
                }
                n40 = call "sync_and_trig_p2p.vi"("error out 2"=w108, "secnario config"=w109) -> ("error out"=w105:errorcluster, "secnario config 2"=w106:T9)  [unwired: 8 in]
              }
            }
            n41 = while {
              tunnel: [w129] -> w27
              tunnel: w29 -> [w138]
              tunnel: [w126] -> w21
              tunnel: w30 -> [w128]
              stop <- w136 stop-if-true
              # "transmit"
              n42 = Unbundle By Name(w128) -> ("mode"=w127:u8)
              n43 = case shown="3" w127 {
                tunnel: w138 -> [w145 w166 w180 w195]
                tunnel: [w139 w164 w178 w193] -> w137
                tunnel: [w142 w163 w177 w192] -> w134
                tunnel: [w143 w162 w176 w191] -> w133
                tunnel: [w144 w160 w174 w189] -> w130
                tunnel: [w140 w158 w172 w187] -> w129
                tunnel: [w141 w157 w171 w186] -> w126
                tunnel: w128 -> [w146 w153 w167 w182]
                frame 0, Default {
                  n44 = call "fpga status 1 ch.vi"("secnario config"=w146, "error in (no error)"=w145) -> ("secnario config"=w150:T9, "fpga clock"=w144:dbl[], "dds free"=w142:bool[][], "pulse transmitted"=w143:u32[], "error out"=w149:errorcluster)  [unwired: 9 in]
                  n45 = And Array Elements(Boolean array=w142) -> (logical AND=w148:bool)
                  n46 = call "write_pulse_1_ch per device_USRP.vi"("error in"=w149, "first call"=FALSE, "secnario config"=w150) -> ("error out"=w141:errorcluster, "num of pulse sent to fpga"=w151:i32, "done write files"=w152:bool, "output cluster"=w140:T9)  [unwired: 4 in, 1 out]
                  n47 = call "done Tx scenario.vi"("all dds free"=w148, "done write files"=w152, "num of pulse sent to fpga"=w151, "pulse transmitted"=w143) -> ("Checkbox out"=w139:bool)  [unwired: 11 in]
                }
                frame 1 {
                  n48 = call "fpga status 5785 2 ch.vi"("secnario config"=w153, "error in (no error)"=w166) -> ("secnario config"=w159:T9, "fpga clock"=w160:dbl[], "dds free"=w163:bool[][], "pulse transmitted"=w162:u32[], "error out"=w161:errorcluster)  [unwired: 9 in]
                  n49 = And Array Elements(Boolean array=w163) -> (logical AND=w165:bool)
                  n50 = call "write_pulse_1_ch per device_1.vi"("error in"=w161, "first call"=FALSE, "secnario config"=w159) -> ("error out"=w157:errorcluster, "num of pulse sent to fpga"=w156:i32, "done write files"=w154:bool, "output cluster"=w158:T9)  [unwired: 4 in, 1 out]
                  n51 = call "done Tx scenario.vi"("all dds free"=w165, "done write files"=w154, "num of pulse sent to fpga"=w156, "pulse transmitted"=w162) -> ("Checkbox out"=w164:bool)  [unwired: 11 in]
                }
                frame 2 {
                  n52 = call "fpga status 5785 1 ch.vi"("secnario config"=w167, "error in (no error)"=w180) -> ("secnario config"=w173:T9, "fpga clock"=w174:dbl[], "dds free"=w177:bool[][], "pulse transmitted"=w176:u32[], "error out"=w175:errorcluster)  [unwired: 9 in]
                  n53 = And Array Elements(Boolean array=w177) -> (logical AND=w179:bool)
                  n54 = call "write_pulse_1_ch per device_1.vi"("error in"=w175, "first call"=FALSE, "secnario config"=w173) -> ("error out"=w171:errorcluster, "num of pulse sent to fpga"=w170:i32, "done write files"=w168:bool, "output cluster"=w172:T9)  [unwired: 4 in, 1 out]
                  n55 = call "done Tx scenario.vi"("all dds free"=w179, "done write files"=w168, "num of pulse sent to fpga"=w170, "pulse transmitted"=w176) -> ("Checkbox out"=w178:bool)  [unwired: 11 in]
                }
                frame 3 {
                  n56 = call "fpga status vst p2p.vi"("secnario config"=w182, "error in (no error)"=w195) -> ("lost sampels"=→"lost sampels":u32, "secnario config"=w188:T9, "fpga clock"=w189:dbl[], "dds free"=w192:bool[][], "pulse transmitted"=w191:u32[], "error out"=w190:errorcluster)  [unwired: 8 in]
                  n57 = And Array Elements(Boolean array=w192) -> (logical AND=w194:bool)
                  n58 = call "write_pulse_1_ch per device_1.vi"("error in"=w190, "first call"=FALSE, "secnario config"=w188) -> ("error out"=w186:errorcluster, "num of pulse sent to fpga"=w185:i32, "done write files"=w183:bool, "output cluster"=w187:T9)  [unwired: 4 in, 1 out]
                  n59 = call "done Tx scenario.vi"("all dds free"=w194, "done write files"=w183, "num of pulse sent to fpga"=w185, "pulse transmitted"=w191) -> ("Checkbox out"=w193:bool)  [unwired: 11 in]
                }
              }
              "clocks" <- w130
              "pulse transmitted" <- w133
              "dds free" <- w134
              n60 = property on="Tab Control" class="TabCtl (strict)"() -> ("Value"=w132:T1)  [unwired: 2 in, 2 out]
              n61 = Not Equal?(x=w132, y=T1."transmit") -> (x != y?=w131:bool)
              n62 = Compound Arithmetic op=OR(w131, invert "run 2", w126, w137) -> (w136:bool)
            }
            n63 = property on="run it again when done" class="Bool (strict)"(error in=w21) -> (error out=w25:errorcluster, "Value"=w23:bool)  [unwired: 1 in, 1 out]
            n64 = Unbundle By Name(w27) -> ("mode"=w26:u8)
            n65 = property on="run 2" class="Bool (strict)"(error in=w21) -> (error out=w20:errorcluster, "Value"=w24:bool)  [unwired: 1 in, 1 out]
            n66 = case shown="3" w26 {
              tunnel: w25 -> [w36 w40 w44]
              tunnel: [w35 w38 w43] -> w32
              tunnel: w27 -> [w34 w39 w42]
              tunnel: [w33 w37 w41] -> w19
              frame 1, 2, Default {
                n67 = call "close all.vi"("error in (no error)"=w36, "secnario config in"=w34) -> ("error out"=w35:errorcluster, "secnario config"=w33:T9)  [unwired: 8 in]
              }
              frame 3 {
                n68 = call "close all p2p.vi"("error in (no error)"=w40, "secnario config in"=w39) -> ("error out"=w38:errorcluster, "secnario config"=w37:T9)  [unwired: 8 in]
              }
              frame 0 {
                n69 = call "close all_ usrp.vi"("error in (no error)"=w44, "secnario config in"=w42) -> ("error out"=w43:errorcluster, "secnario config in 2"=w41:T9)  [unwired: 8 in]
              }
            }
            n70 = And(x=w23, y=w24) -> (x .and. y?=w22:bool)
            n71 = property on="run 2" class="Bool (strict)"(error in=w32, "Value"=w22) -> (error out=w31:errorcluster)  [unwired: 1 in, 1 out]
          }
        }
      }
      frame "scenario generate", "file setup", Default {
        n72 = event shown="[1] \"generate\": Value Change" {
          selector: _ -> [_ _ _ _]
          dyn-events: _ -> [_ _ _ _]
          timeout: 50 -> [_ _ _ _]
          tunnel: [w209 w224 w247 _] -> w200
          tunnel: w198 -> [w212 w223 w252 w271]
          tunnel: "gen for DF" -> [_ w227 w251 _]
          tunnel: [w203 w222 w250 w270] -> w199
          tunnel: w197 -> [_ _ _ w267]
          event "refresh_file show": Value Change {
            # "used for closeing all the TDMS files"
            n73 = event-data() -> ()  [unwired: 1 in, 1 out]
            n74 = call "ini_file_read_pulse_tx.vi"("secnario config"=w212) -> ("error out"=w211:errorcluster, "output cluster"=w208:T9)  [unwired: 9 in]
            n75 = call "collect pulses.vi"("error in (no error)"=w211, "max number of pulses to show"="max number of pulses to show", "time range"="time range", "secnario config"=w208) -> ("error out"=w210:errorcluster, "PDW"=w204:cluster{"PDW":T19[], "Ton":dbl[]}, "secnario config"=w206:T9)  [unwired: 5 in]
            n76 = call "close all.vi"("error in (no error)"=w210, "secnario config in"=w206) -> ("error out"=w209:errorcluster, "secnario config"=w203:T9)  [unwired: 8 in]
            n77 = call "pdw 2 graph.vi"("color plate"="color plate", "PDW"=w204, "secnario config"=w203) -> ("color"=w214:u32[], "graph"=w202:cluster{dbl[], dbl[]}[])  [unwired: 7 in]
            n78 = flat-sequence {
              tunnel: w214 -> [w217]
              tunnel: [w217] -> w213
              tunnel: w202 -> [w216]
              tunnel: w213 -> [w218]
              frame #0 {
                "XY Graph" <- w216
              }
              frame #1 {
                n79 = for {
                  tunnel: w218 -> [w220] mode=indexing
                  i -> [w219]
                  n80 = property on="XY Graph" class="XYGraph (strict)"("Active Plot"=w219, "Plot.Plot Color"=w220) -> ()  [unwired: 2 in, 2 out]
                }
              }
            }
          }
          event "generate": Value Change {
            # "PDW- \nsorted by time"
            n81 = event-data() -> ()  [unwired: 1 in, 1 out]
            n82 = call "gen random emmiters.vi"("rand limits"="rand limits", "secnario config"=w223) -> ("Array"=w239:T6[])  [unwired: 9 in]
            n83 = Unbundle By Name(w223) -> ("center frequency (Hz)"=w232:dbl, "Fs  FPGA"=w231:dbl, "SPC"=w230:dbl, "file paths"=w229:path[])
            n84 = Build Array (concatenate)("user bulid emitters", w239) -> (w236:T6[])
            n85 = call "emitters to PDWs.vi"("emmiter"=w236, "center frequency (Hz)"=w232) -> ("sorted array"=w238:T20[], "erorr out"=w235:errorcluster)  [unwired: 11 in, 1 out]
            n86 = Array Size(array=w238) -> (size(s)=→"num of pulses":i32)
            n87 = call "pdw to raw PDW.vi"("PDWs"=w238, "Fs fpGa"=w231, "SPC"=w230, "gen for DF"=w227, "erorr in"=w235) -> ("Array"=w233:u64[][], "erorr out"=w234:errorcluster)  [unwired: 8 in, 1 out]
            n88 = for {
              tunnel: w229 -> [w244]
              tunnel: w233 -> [w246] mode=indexing
              tunnel: [w241] -> w226 mode=indexing
              shift-right: [w245] -> w225
              shift-left: w234 -> [w242]
              i -> [w243]
              # "write PDWs to TDMS file"
              n89 = call "get a name.vi"("error constant"=w242, "Numeric"=w243, "tdms pulse istraction file in"=w244) -> ("error constant 2"=w240:errorcluster, "Path"=w241:path)  [unwired: 7 in]
              n90 = call "data to file.vi"("error in (no error)"=w240, "Array"=w246, "Path"=w241) -> ("error out"=w245:errorcluster)  [unwired: 8 in]
            }
            n91 = Bundle By Name(cluster=w223, "file paths"=w226) -> (w222:T9)
            n92 = property on="file paths" class="Arr (strict)"(error in=w225, "Value"=w226) -> (error out=w224:errorcluster)  [unwired: 1 in, 1 out]
          }
          event "convert Button": Value Change {
            n93 = event-data() -> ()  [unwired: 1 in, 1 out]
            n94 = Unbundle By Name(w252) -> ("file paths"=w254:path[], "center frequency (Hz)"=w257:dbl, "Fs  FPGA"=w256:dbl, "SPC"=w255:dbl)
            n95 = call "csv_to PDW.vi"("CSV file path (dialog if empty)"="csv pulse istraction file in", "Fbase"=w257, "Fs"=w256, "gen for DF"=w251, "SPC"=w255) -> ("u64_PDW"=w259:u64[][], "error out"=w258:errorcluster)  [unwired: 9 in]
            n96 = for {
              tunnel: w254 -> [w266]
              tunnel: w259 -> [w261] mode=indexing
              tunnel: w258 -> [w264]
              tunnel: [w260] -> w249 mode=indexing
              tunnel: [w262] -> w248
              i -> [w265]
              n97 = call "get a name.vi"("error constant"=w264, "Numeric"=w265, "tdms pulse istraction file in"=w266) -> ("error constant 2"=w263:errorcluster, "Path"=w260:path)  [unwired: 7 in]
              n98 = call "data to file.vi"("error in (no error)"=w263, "Array"=w261, "Path"=w260) -> ("error out"=w262:errorcluster)  [unwired: 8 in]
            }
            n99 = Bundle By Name(cluster=w252, "file paths"=w249) -> (w250:T9)
            n100 = property on="file paths" class="Arr (strict)"(error in=w248, "Value"=w249) -> (error out=w247:errorcluster)  [unwired: 1 in, 1 out]
          }
          event Timeout; "user configurations.Dial", "user configurations.center frequency (Hz)", "user configurations.buffer size", "user configurations.devicess", "user configurations.RF gain", "user configurations.file paths": Value Change {
            n101 = event-data() -> ()  [unwired: 1 in, 1 out]
            n102 = call "update config.vi"("user configurations"=w267, "secnario config in"=w271) -> ("Numeric"=w268:dbl, "Numeric 2"=w269:dbl, "secnario config out"=w270:T9)  [unwired: 7 in]
            n103 = property on="f band range" class="Slide (strict)"("Scale.Maximum"=w269, "Scale.Minimum"=w268) -> ()  [unwired: 2 in, 2 out]
          }
        }
      }
    }
    n104 = Or(x=w2, y="end program") -> (x .or. y?=w7:bool)
    n105 = call <vilib>:"Simple Error Handler.vi"("error in (no error)"=w2) -> ()  [unwired: 4 in, 5 out]
  }
